vi "02 HEWH_RLTTesting_SM.vi"() -> ()   [LabVIEW 2011]
uses:
  <vilib>/Platform/fileVersionInfo.llb/FileVersionInformation.ctl
  PowerElements.ctl
  Intellifaucet/Intellfaucet Mode.ctl
  ValveBankPositions.ctl
  TestedFlowratesScenarios.ctl
  EquipReferences.ctl
  HEWH Error Enumeration.ctl
  Global HEWH.vi
panel:
  in  "Test Tank":string="101,102,103,104,105,106,107,108,109,110,111,112,113,114,115,116"
  out "Error Count":dbl
  out "result 4":bool
  out "result 3":bool
  out "result 2":bool
  out "result":bool
  out "Draws Left":i32
  out "FileNameD":path caption="FileName"
  out "FileNameC":path caption="FileName"
  out "FileNameB":path caption="FileName"
  in  "Tab Control":T1(tab)=enum."RLT Control"
  out "FileVersionInfo Out":T2
  in  "End Test":bool
  out "Finish":bool=TRUE
  out "Stop Logging":bool=TRUE
  in  "RLT Equipment":T3={"COM A"="COM3", "MW100"="MW100", "AG34970"="A-34972A", "COM B"="COM4", "COM C"="COM5", "COM D"="COM6"}
  out "Local?":bool
  out "DataQ":refnum<queue>
  in  "Flow Setting(GPM)":dbl=3.0
  in  "Temp Band":dbl=2.0
  out "Stopped Serial A":bool=TRUE
  out "Stopped Serial B":bool=TRUE
  out "Stopped Serial C":bool=TRUE
  out "Stopped Serial D":bool=TRUE
  in  "Expansion Tank?":bool=TRUE
  out "Test Started":bool=TRUE
  out "Station D Channels, Agilent":string[](array[string])
  out "Station B Channels, Agilent":string[](array[string])
  out "Station A Channels, Agilent":string[](array[string])
  out "Station C Channels, Agilent":string[](array[string])
  out "Station C Channels, MW100":string[](array[string])
  out "Station D Channels, MW100":string[](array[string])
  out "Station B Channels, MW100":string[](array[string])
  out "Station A Labels, MW100":string[](array[string])
  out "Station A Labels, Agilent":string[](array[string])
  out "Station B Labels, Agilent":string[](array[string])
  out "Station B Labels, MW100":string[](array[string])
  out "Station C Labels, Agilent":string[](array[string])
  out "Station C Labels, MW100":string[](array[string])
  out "Station D Labels, Agilent":string[](array[string])
  out "Station D Labels, MW100":string[](array[string])
  out "Station A Channels, MW100":string[](array[string])
  in  "Agilent Scan List":string="101,102,103,104,105,106,107,108,109,110,111,112,113,114,115,116"
  out "Versions":string[](array[string])
  out "Error Log":errorcluster[](array[cluster])
  in  "Gather Data Period":i32=10000
  out "Computer Name":string
  out "FileNameA":path=path "c:/data/20110112-2122_HEWH-MAN_OV.csv"
  in  "Work File Directory":path=path "c:/Work"
  out "IP Add":string
  in  "Save File Directory":path=path "c:/Data"
  in  "Divisor":i32=2000
  out "HEWH Sample Rate":i32=10
  out "T1 ComTimer":i32=1000
  in  "FlowPoll Rate":i32=10
  out "MW100 Data":dbl[](array[numeric]) format="%.4f"
  out "Agilent Output Data":dbl[](array[numeric])
  in  "MW100 Semiphore":T4=refnum
  out "Serial Data A":string[][](array[string])
  out "Serial Data B":string[][](array[string])
  out "Serial Data C":string[][](array[string])
  out "Serial Data D":string[][](array[string])
  out "A Data Array":string[][](array[string])
  out "B Data Array":string[][](array[string])
  out "C Data Array":string[][](array[string])
  out "D Data Array":string[][](array[string])
  out "# elements in queue":i32
  out "Count A":dbl
  out "Count B":dbl
  out "Count C":dbl
  out "Count D":dbl
  out "UI Update Loop":i32
  out "No Draw D":bool
  out "No Draw C":bool
  out "No Draw B":bool
  out "No Draw A":bool
  out "ComD":bool
  out "ComC":bool
  out "ComB":bool
  in  "Current Draw(D)":i32
  in  "Current Draw(C)":i32
  out "POWERC":T5
  out "POWERD":T5
  out "Alarm C":bool
  out "Alarm D":bool
  out "Alarm A":bool
  in  "Current Draw(A)":i32
  out "ComA":bool
  out "POWERA":T5
  out "POWERB":T5
  out "Alarm B":bool
  in  "Current Draw(B)":i32
  out "Drawing":bool
  in  "Start Test":bool
  in  "Num Draws (D)":i32
  in  "Num Draws (C)":i32
  in  "Num Draws (B)":i32
  out "Draw Amount (GAL)":dbl=15.0
  in  "Num Draws (A)":i32
  in  "Thermal Limit":dbl=260.0
  in  "EEV Limit":dbl=500.0
  out "Com Setting":bool=TRUE
  out "Elapsed Time":dbl format="%<%H:%M:%S>t"
  out "InitOK":bool
  out "M*(Gal)":dbl
  out "Flow":dbl=3.8899999999999997
  out "Status Message":string
  in  "Stop Test Now":bool
  out "Test States":string[](array[string])
  out "Degree Setting(F)":dbl=58.0
  out "UI":bool
  out "Tc_down":dbl
  out "Ver.":string="Development"
  in  "Pause test":bool
  out "Downspout Flow Chart":dbl(graph)=2.9
  out "Downspout Temp Chart":dbl(graph)=57.8
  out "Flow Out":dbl
  in  "K(0.2)":dbl=0.2
  out "Temp Control Sig":dbl=61.459999999999994
  out "Init Complete":bool
  out "error out":errorcluster
  # "="
  # "Gather Data Period is how often data is gathered (roughtly)\nHEWH Sample Rate is how often the serial ports are polled in GEA2.  The latest data is saved in the file.\nT1 ComTimer is the delay used through the test in the loops.\nFlow Poll Rate is how often the flow is polled (number of T1 ComTimer cycles) during Wait for Power Off."
  # "ms per cycle"
  # "HEWH RLT TEST"
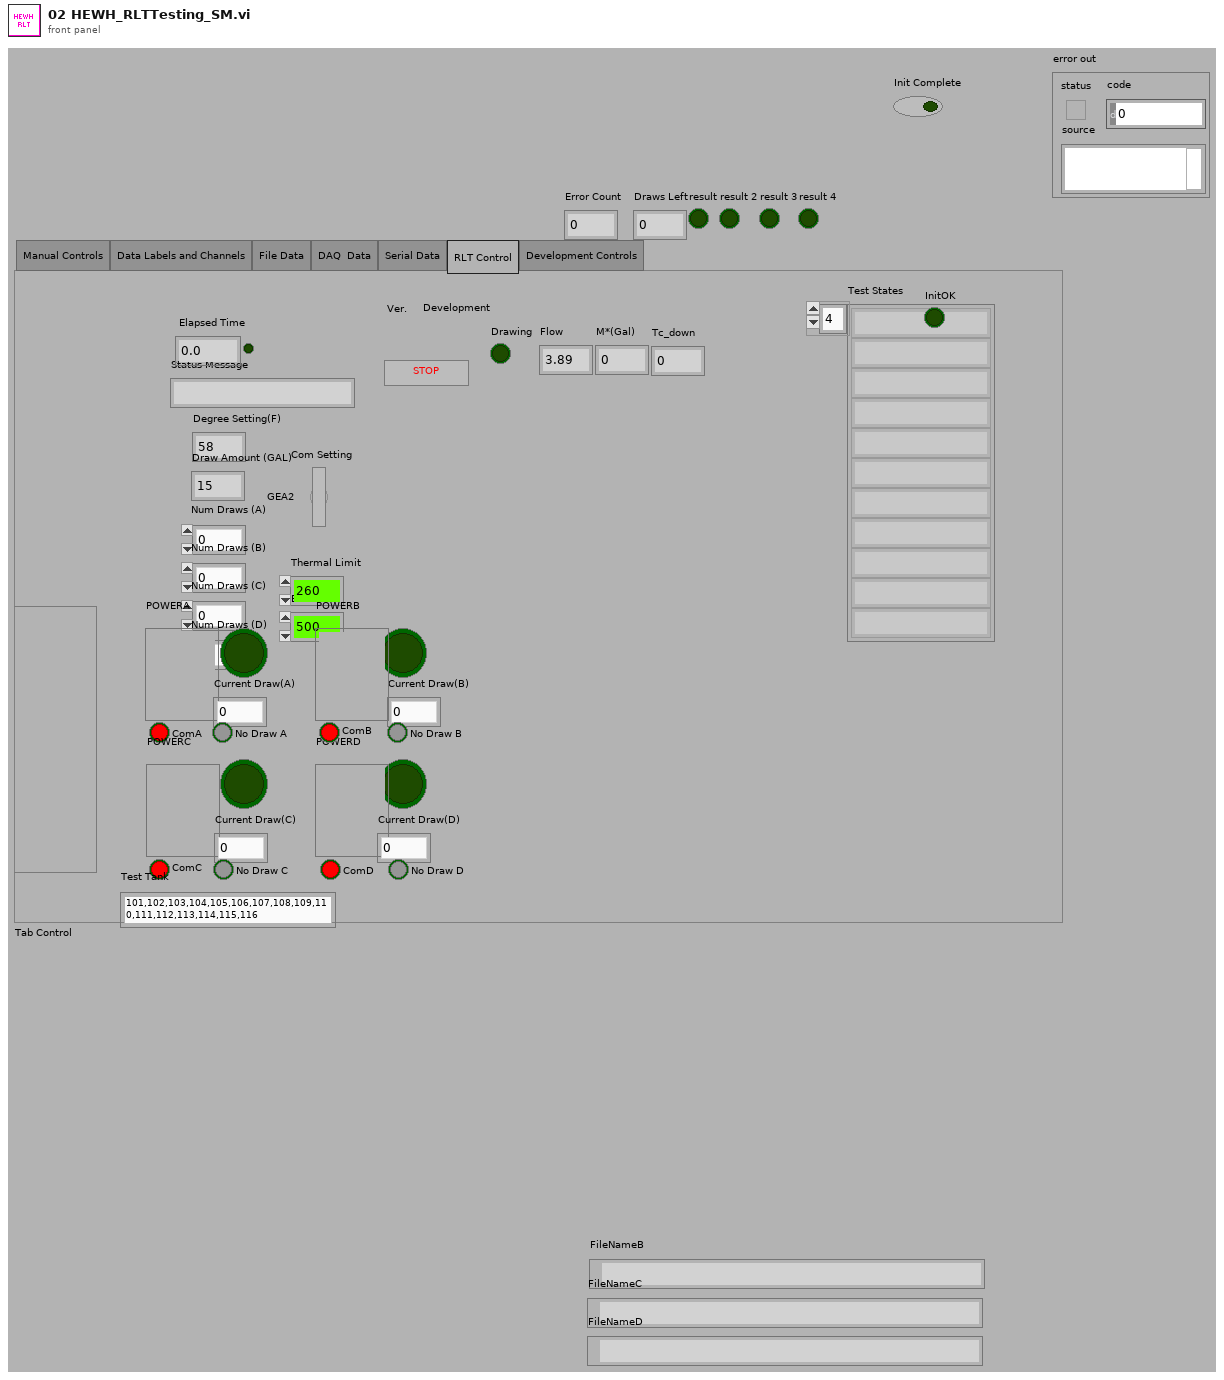
[diagram p1: front panel]
types:
  T1 = enum32{"Manual Controls", "Data Labels and Channels", "File Data", "DAQ  Data", "Serial Data", "RLT Control", "Development Controls"}
  T2 = typedef "FileVersionInformation.ctl" = cluster{"FileVersion":string, "ProductName":string, "InternalName":string, "CompanyName":string, "LegalCopyright":string, "FileDescription":string}
  T3 = cluster{"COM A":refnum<visa-resource-name>, "MW100":refnum<visa-resource-name>, "AG34970":refnum<visa-resource-name>, "COM B":refnum<visa-resource-name>, "COM C":refnum<visa-resource-name>, "COM D":refnum<visa-resource-name>}
  T4 = typedef "Semaphore RefNum" = refnum<k1>
  T5 = typedef "PowerElements.ctl" = cluster{"UE":bool, "LE":bool, "COMP":bool, "FANS":bool}
  T6 = cluster{"Degree Setting(F)":dbl, "Com Setting":bool, "EEV Limit":dbl, "Thermal Limit":dbl, "Num Draws (A)":i32, "Draw Amount (GAL)":dbl, "Num Draws (B)":i32, "Num Draws (C)":i32, "Num Draws (D)":i32}
  T7 = enum32{"invalid app kind", "Development System", "Run Time System", "Student Edition", "Embedded LabVIEW", "Evaluation", "Custom"}
  T8 = typedef "ValveBankPositions.ctl" = enum16{"Heating", "Purge", "Resting", "Draw"}
  T9 = typedef "Intellfaucet Mode.ctl" = enum16{"Adjust Temp", "Adjust Flow", "Start Flow", "Stop Flow"}
  T10 = enum32{"Invalid", "Standard", "Closed", "Hidden", "Minimized", "Maximized"}
  T11 = enum16{"Computation Start", "Computation stop", "Reset Computation", "Clear Computation"}
  T12 = typedef "TestedFlowratesScenarios.ctl" = enum16{"DRK500,Station1", "DRK375,Lab", "SRK500,Station1,5GPM FR", "DRK375,STATION3,1/2\"HOSE", "DRK500,Station1,downspout", "DRK375,Station3,thruEcocute", "DRK375,Station3,purge", "Build2,2B,Purge", "Global, Purge", "Global, Tank"}
  T13 = typedef "EquipReferences.ctl" = cluster{"COM Port":refnum<visa-resource-name>, "MW100":refnum<visa-resource-name>, "AG34970":refnum<visa-resource-name>, "Chamber":refnum<visa-resource-name>}
  T14 = typedef "HEWH Error Enumeration.ctl" = enum16{"No Error", "GEA2 Send ACK Mismatch", "GEA2 STX", "GEA2 ETX", "GEA2 CRC Mismatch", "GEA2 ReadACK", "RTD In Range Error", "Fail Mean Tank Temp", "No Flow Config Data Found", "Failed Flow During Purge", "Temp During Purge", "Confirm IF Stop Fail", "Init Draw: TC_1 Out of Range", "Flow = 0 During Draw after 20s"}
  T15 = cluster{"Core":cluster{"Current VI Reference":refnum<vi>, "Close Panel on Exit?":bool}, "RLT Equipment":cluster{"COM A":refnum<visa-resource-name>, "MW100":refnum<visa-resource-name>, "AG34970":refnum<visa-resource-name>, "COM B":refnum<visa-resource-name>, "COM C":refnum<visa-resource-name>, "COM D":refnum<visa-resource-name>}, "semaphore":T4, "Agilent Scan List":string, "Degree Setting(F)":dbl, "Flow Setting(GPM)":dbl, "Local?":bool, "Com Setting":bool, "Temp Band":dbl, "DrawsLeft":i32[], "Error Log":errorcluster[], "Test Tank":string}
  T16 = typedef "RLT Stations.ctl" = cluster{"MW100 Labels_Channels":T17[], "Agilent Labels_Channels":T17[]}
  T17 = typedef "LabelChannel.ctl" = cluster{"Label":string, "Channel":string}
  T18 = cluster{"Current VI Reference":refnum<vi>, "Close Panel on Exit?":bool}
  T19 = cluster{"MW100 Data":dbl[], "Serial Data A":string[][], "Serial Data A":string[][], "Serial Data A":string[][], "Serial Data A":string[][], "MW100 Data":dbl[]}
  T20 = cluster{"Alarm A":bool, "Current Draw(A)":i32, "ComA":bool, "POWER":T5}
  T21 = cluster{"MW100 Data":dbl[], "Serial Data A":string[][], "Serial Data B":string[][], "Serial Data C":string[][], "Serial Data D":string[][], "Agilent Output Data":dbl[]}
  T22 = cluster{"Q Element":cluster{"MW100 Data":dbl[], "Serial Data A":string[][], "Serial Data B":string[][], "Serial Data C":string[][], "Serial Data D":string[][], "Agilent Output Data":dbl[]}, "A Data Array":string[][], "B Data Array":string[][], "C Data Array":string[][], "D Data Array":string[][], "RLT Tank A":cluster{"Alarm A":bool, "Current Draw(A)":i32, "ComA":bool, "POWER":T5}, "RLT Tank B":cluster{"Alarm A":bool, "Current Draw(A)":i32, "ComA":bool, "POWER":T5}, "RLT Tank C":cluster{"Alarm A":bool, "Current Draw(A)":i32, "ComA":bool, "POWER":T5}, "RLT TankD":cluster{"Alarm A":bool, "Current Draw(A)":i32, "ComA":bool, "POWER":T5}}
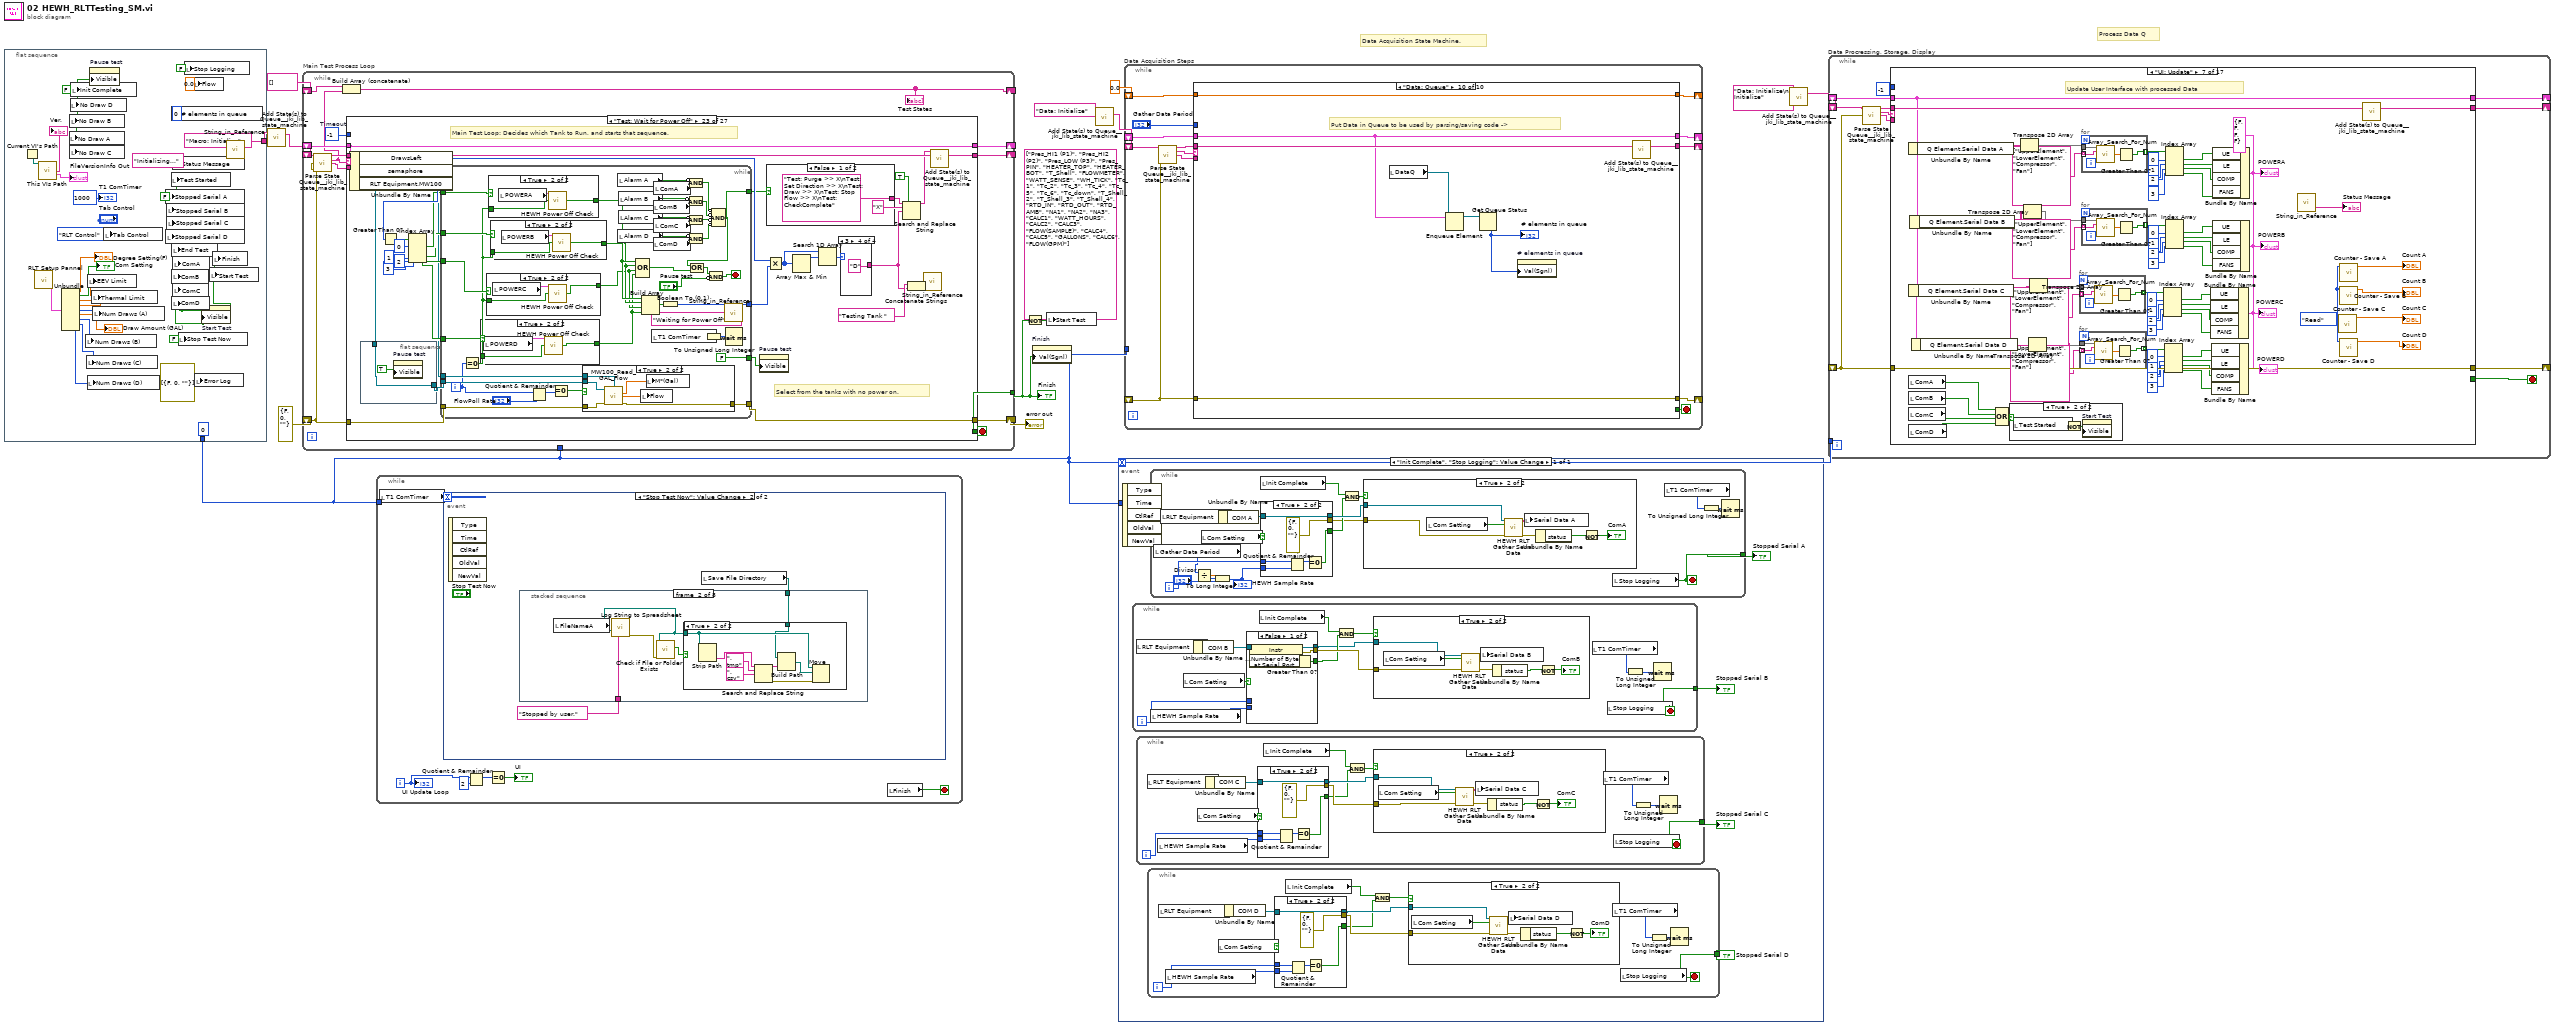
[diagram p0: block diagram]
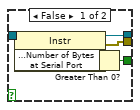
[diagram p2: hidden frame]
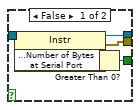
[diagram p4: hidden frame]
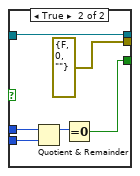
[diagram p6: hidden frame]
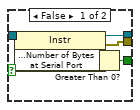
[diagram p8: hidden frame]
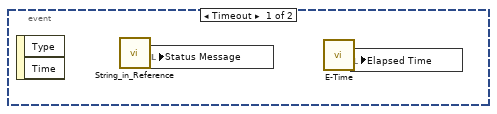
[diagram p10: hidden frame]
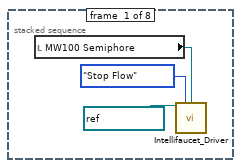
[diagram p11: hidden frame]
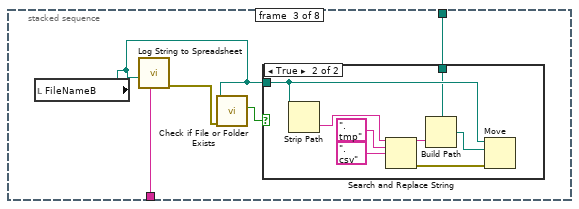
[diagram p13: hidden frame]
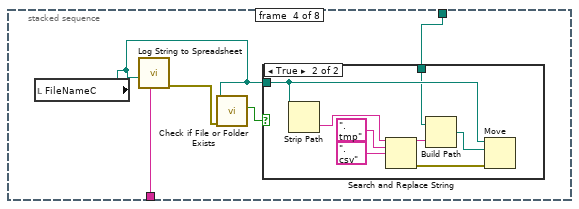
[diagram p15: hidden frame]
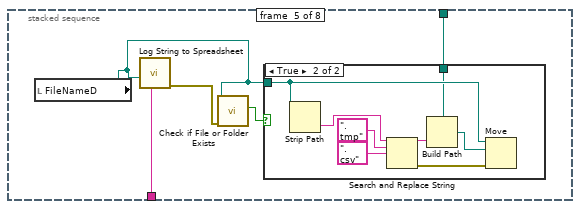
[diagram p17: hidden frame]
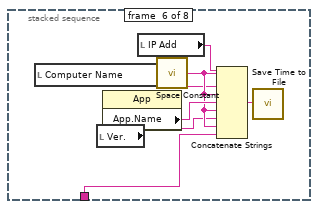
[diagram p19: hidden frame]
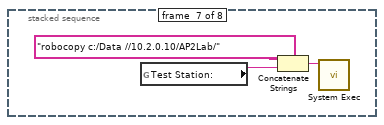
[diagram p20: hidden frame]
diagram:
  (unwired) string[] ["Pres_HI1 (P1)", "Pres_HI2 (P2)", "Pres_LOW (P3)", "Pres_PIN", "HEATER_TOP", "HEATER_BOT", "T_Shell", "FLOWMETER", "WATT_SENSE", "WH_TICK", "Tc_1", "Tc_2", "Tc_3", "Tc_4", "Tc_5", "Tc_6", "Tc_down", "T_Shell_2", "T_Shell_3", "T_Shell_4", "RTD_IN", "RTD_OUT", "RTD_AMB", "NA1", "NA2", "NA3", "CALC1", "WATT_HOURS", "CALC2", "CALC3", "FLOW(SAMPLE)", "CALC4", "CALC5", "GALLONS", "CALC6", "FLOW(GPM)"] ("output array")
  # "Process Data Q"
  # "Data Acquisition State Machine."
  n1 = flat-sequence {
    tunnel: ["Macro: Initialize"] -> w7
    tunnel: [0 ("T1 ComTimer")] -> w4
    frame #0 {
      w30 = "Initializing..." ("String")
      w14 = FALSE ("Stopped Serial A")
      w15 = FALSE ("Init Complete")
      n2 = Current VI's Path() -> (path=w18:path)
      n3 = call "RLT Setup Pannel.vi"() -> ("RLT Setup Out"=w28:T6)  [unwired: 15 in]
      n4 = call "This VIs Path.vi"("path"=w18) -> ("File Version Info"=→"Ver.":string, "FileVersionInfo Out"=→"FileVersionInfo Out":T2)  [unwired: 10 in, 3 out]
      n5 = Unbundle(w28) -> ("Degree Setting(F)"=→"Degree Setting(F)":dbl, "Com Setting"=→"Com Setting":bool, "EEV Limit"=w21:dbl, "Thermal Limit"=w20:dbl, "Num Draws (A)"=w24:i32, "Draw Amount (GAL)"=→"Draw Amount (GAL)":dbl, "Num Draws (B)"=w23:i32, "Num Draws (C)"=w22:i32, "Num Draws (D)"=w19:i32)
      n6 = local write "No Draw A"(w15) -> ()
      n7 = local write "No Draw B"(w15) -> ()
      n8 = local write "No Draw C"(w15) -> ()
      n9 = local write "No Draw D"(w15) -> ()
      n10 = local write "Init Complete"(w15) -> ()
      n11 = local write "Num Draws (B)"(w23) -> ()
      n12 = local write "Num Draws (C)"(w22) -> ()
      n13 = local write "Num Draws (D)"(w19) -> ()
      n14 = local write "EEV Limit"(w21) -> ()
      n15 = property on="Pause test" class="Bool (strict)"("Visible"=w15) -> ()  [unwired: 2 in, 2 out]
      n16 = local write "Thermal Limit"(w20) -> ()
      n17 = local write "Num Draws (A)"(w24) -> ()
      n18 = local write "Tab Control"(T1."RLT Control" ("Tab Control")) -> ()
      n19 = local write "Stopped Serial A"(w14) -> ()
      n20 = local write "Stopped Serial D"(w14) -> ()
      n21 = local write "Stopped Serial B"(w14) -> ()
      n22 = local write "Stopped Serial C"(w14) -> ()
      n23 = local write "Test Started"(w14) -> ()
      n24 = local write "# elements in queue"(0 ("# elements in queue")) -> ()
      n25 = local write "End Test"(w14) -> ()
      n26 = local write "ComB"(w14) -> ()
      n27 = local write "ComD"(w14) -> ()
      n28 = local write "Status Message"(w30) -> ()
      n29 = local write "ComA"(w14) -> ()
      n30 = local write "ComC"(w14) -> ()
      n31 = local write "Stop Test Now"(FALSE ("Stop Test Now")) -> ()
      n32 = local write "Stop Logging"(FALSE ("Stop Logging")) -> ()
      n33 = local write "Flow"(0.0 ("Flow")) -> ()
      n34 = local write "Error Log"(errorcluster[] [{"status"=FALSE, "code"=0, "source"=""}] ("Error Log")) -> ()
      n35 = property on="Start Test" class="Bool (strict)"("Visible"=w14) -> ()  [unwired: 2 in, 2 out]
      n36 = local write "Start Test"(w14) -> ()
      n37 = local write "Finish"(w14) -> ()
      n38 = call "String_in_Reference.vi"("String"=w30) -> ()  [unwired: 18 in, 1 out]
      "T1 ComTimer" <- 1000 ("T1 ComTimer")
    }
  }
  n39 = call <vilib>:"Add State(s) to Queue__jki_lib_state_machine.vi"("State(s) at Back (\"\")"=w7) -> ("States Out"=w13:string)  [unwired: 14 in]
  n40 = while "Main Test Process Loop" {
    shift-right: [w47] -> _
    shift-left: _ -> [w46]
    shift-right: [w49] -> w12
    shift-left: errorcluster {"status"=FALSE, "code"=0, "source"=""} ("Error Out") -> [w44]
    shift-right: [w48] -> _
    shift-left: w13 -> [w50]
    tunnel: [w43] -> w1
    shift-right: [w42] -> _
    shift-left: string[] [] -> [w41]
    tunnel: w4 -> [_]
    stop <- w43 stop-if-true
    w45 = -1  # Timeout
    n41 = call <vilib>:"Parse State Queue__jki_lib_state_machine.vi"("State Queue"=w50, "Error In (no error)"=w44) -> ("Remaining States"=w51:string, "Current State"=w39:string, "Arguments"=w40:string)  [unwired: 11 in]
    n42 = Build Array (concatenate)(w41, w39) -> (w42:string[])
    "Test States" <- w42
    n43 = case shown="\"Test: Wait for Power Off\"" w39 {
      selector: w39 -> [_ _ w108 _ _ _ _ _ _ _ _ _ _ _ _ _ _ _ _ _ _ w471 _ _ _ _ _]
      tunnel: w51 -> [w58 w107 w112 w130 w150 w241 w287 w306 w326 w359 w371 w390 w396 w400 w406 w412 w423 w449 w454 w465 w469 w496 w545 w634 w671 w706 w753]
      tunnel: w40 -> [_ _ _ _ _ _ _ _ _ _ _ _ _ _ _ w407 w417 _ _ _ _ _ _ w626 w666 w680 w736]
      tunnel: w46 -> [w56 w104 w110 w121 w133 w238 w275 w303 w322 w355 w368 _ w391 w397 w404 w410 w419 w446 w451 w462 w466 w489 w542 w632 w669 w704 w749]
      tunnel: [w55 w105 w114 w127 w148 w225 w267 w304 errorcluster {"status"=FALSE, "code"=0, "source"=""} ("error out") w347 w369 w380 w392 w398 w403 w408 w420 w447 w452 w463 w467 w494 w519 w618 w665 w688 w741] -> w49
      tunnel: w44 -> [w54 w105 w113 w127 w148 w239 w265 w304 w319 w356 w369 w381 w393 w398 w403 w409 w421 w447 w452 w463 w467 w494 w520 w625 w664 w691 w747]
      tunnel: [w57 w106 w111 w129 w149 w240 w286 w305 w325 w358 w370 w389 w395 w399 w405 w411 w422 w448 w453 w464 w468 w495 w544 w633 w670 w705 w752] -> w48
      tunnel: [_ _ _ _ _ _ _ _ _ TRUE _ _ _ _ _ _ _ _ _ _ _ _ _ _ _ _ _] -> w43
      tunnel: [w53 w104 w110 w128 w132 w237 w275 w303 w321 w355 w368 w388 w391 w397 w404 w410 w419 w446 w451 w462 w466 w488 w542 w632 w669 w704 w749] -> w47
      tunnel: w45 -> [w52 _ _ _ _ _ _ _ _ _ _ _ _ _ _ _ _ _ _ _ _ _ _ _ _ _ _]
      frame "", "Idle" {
        # "executes when the state queue is empty"
        n44 = event shown="[2] \"Start Test\": Value Change" {
          selector: _ -> [_ _ _ _]
          dyn-events: _ -> [_ _ _ _]
          timeout: w52 -> [_ _ _ _]
          tunnel: w58 -> [w62 w67 w86 w103]
          tunnel: [w61 w66 w85 w102] -> w57
          tunnel: w56 -> [w59 w64 w83 w100]
          tunnel: [w60 w65 w84 w101] -> w55
          tunnel: w54 -> [w60 w65 w84 w101]
          tunnel: [w59 w64 w83 w100] -> w53
          event Timeout {
            n45 = event-data() -> ()  [unwired: 1 in, 1 out]
            n46 = call <vilib>:"Add State(s) to Queue__jki_lib_state_machine.vi"("State(s) in (\"\")"=w62) -> ("States Out"=w61:string)  [unwired: 14 in]
          }
          event "End Test": Value Change {
            # "Exit Button Value Change (pressed) Event\n(this executes Macro: Exit to terminate the VI)"
            n47 = event-data() -> ()  [unwired: 1 in, 1 out]
            n48 = call <vilib>:"Add State(s) to Queue__jki_lib_state_machine.vi"("State(s) in Front (\"\")"="Macro: Exit", "State(s) in (\"\")"=w67) -> ("States Out"=w66:string)  [unwired: 13 in]
          }
          event "Start Test": Value Change {
            n49 = event-data() -> ()  [unwired: 1 in, 6 out]
            n50 = local read "Num Draws (B)"() -> (w79:i32)
            n51 = local read "Num Draws (D)"() -> (w77:i32)
            n52 = local read "Num Draws (A)"() -> (w80:i32)
            n53 = local read "Num Draws (C)"() -> (w78:i32)
            n54 = local read "FileNameD"() -> (w73:path)
            n55 = local read "FileNameC"() -> (w74:path)
            n56 = local read "FileNameA"() -> (w76:path)
            n57 = local read "FileNameB"() -> (w75:path)
            n58 = call "String_in_Reference.vi"("String"="Starting Test..." ("string")) -> ()  [unwired: 18 in, 1 out]
            n59 = Build Array(w76, w75, w74, w73) -> (w72:path[])
            n60 = Build Array(w80, w79, w78, w77) -> (w71:i32[])
            n61 = for {
              tunnel: w72 -> [w90] mode=indexing
              tunnel: w71 -> [w89] mode=indexing
              tunnel: "Start Test" -> [_]
              tunnel: [FALSE ("Visible")] -> w69
              tunnel: [TRUE] -> w68
              n62 = local read "Draw Amount (GAL)"() -> (w94:dbl)
              n63 = local read "Degree Setting(F)"() -> (w92:dbl)
              n64 = Format Into String(format string="%s %d %s %f %s %f", "Number of Draws: ", w89, " Draw Amount: ", w94, " H2O Temp In Setting: ", w92) -> (resulting string=w91:string)  [unwired: 2 in, 1 out]
              n65 = call "Log String to Spreadsheet.vi"("String"=w91, "FileName"=w90) -> ()  [unwired: 9 in, 1 out]
            }
            "Test Started" <- w68
            n66 = property on="Start Test" class="Bool (strict)"("Visible"=w69) -> ()  [unwired: 2 in, 2 out]
            n67 = call <vilib>:"Add State(s) to Queue__jki_lib_state_machine.vi"("State(s) in Front (\"\")"="Test: CheckComplete", "State(s) in (\"\")"=w86) -> ("States Out"=w85:string)  [unwired: 13 in]
          }
          event Panel Close? {
            # "Discard the event because we'll close the front panel ourselves in Macro: Exit"
            # "Close Panel button (pressed) Event\n(this executes Macro: Exit to terminate the VI)"
            n68 = event-data() -> ()  [unwired: 1 in, 1 out]
            n69 = call <vilib>:"Add State(s) to Queue__jki_lib_state_machine.vi"("State(s) in Front (\"\")"="Macro: Exit", "State(s) in (\"\")"=w103) -> ("States Out"=w102:string)  [unwired: 13 in]
            n70 = event-data("Discard?"=TRUE) -> ()  [unwired: 1 in, 1 out]
          }
        }
      }
      frame "---------- Core ----------" {
        # "Do not put any code in this frame.\n(it is a separator no-op)"
        n71 = call <vilib>:"Add State(s) to Queue__jki_lib_state_machine.vi"("State(s) in (\"\")"=w107) -> ("States Out"=w106:string)  [unwired: 14 in]
      }
      frame Default {
        w117 = 42 items=["No error", "Argument error", "Memory is full", "Out of zone", "End of file", "File already open", "Generic file I/O error", "File not found", "File permission error", "Disk is full", "Duplicate path", "Too many files open", "System feature not enabled", "Resource file not found", "Cannot add resource", "Resource not found", "Image not found", "Image memory error", "Pen does not exist", "Config type invalid", "Config token not found", "Config parse error", "Config memory error", "Bad external code format", "Bad external code offset", "External code not present", "Null window", "Destroy window error", "Null menu", "Print aborted", "Bad print record", "Print driver error", "Windows error during printing", "Memory error during printing", "Print dialog error", "Generic print error", "Invalid device refnum", "Device not found", "Device parameter error", "Device unit error", "Cannot open device", "Device call aborted", "Generic error", "Cancelled by user", "Object ID too low", "Object ID too high", "Object not in heap", "Unknown heap", "Unknown object (invalid DefProc)", "Unknown object (DefProc not in table)", "Message out of range", "Invalid (null) method", "Unknown message", "Manager call not supported", "Bad address", "Network operation in progress", "Network operation timed out", "Connection is busy", "Network attribute not supported", "Network error", "Address in use", "System out of memory", "Connection aborted", "Connection refused", "Not connected", "Already connected", "Connection closed", "Initialization error (interapplication manager)", "Bad occurrence", "Wait on unbound occurrence handler", "Occurrence queue overflow", "Datalog type conflict", "Unused", "Unrecognized type (interapplication manager)", "Memory corrupt", "Failed to make temporary DLL", "Old CIN version", "Drag socket not found", "Failed to load drop-object", "Failed to register OLE object", "Failed to release OLE object", "Format specifier type mismatch", "Unknown format specifier", "Too few format specifiers", "Too many format specifiers", "Scan failed", "Newer CIN version", "Error converting to variant", "Runtime menu error", "Password tampered", "Variant attribute not found", "Incompatible variant data type", "Event data is not available", "Event Store is not present", "Occurrence is not found", "Event Queue is not created", "Event info is not available", "Refnum passed is NULL", "Error retrieving Class GUID", "Error retrieving CoClass GUID", "Error retrieving TypeLib GUID.", "Bad built application magic bytes.", "Specific driver is different from the specific driver associated with the Logical Name.", "There is no session opened to the class driver.", "Max Error", "MAX - Error with config objects", "MAX - Error loading configuration", "MAX - Group not supported"]
        # "Current State"
        # "Do not delete, rename, or modify this frame.\n(this is used to capture unhandled states and typos)"
        # "Handle mistyped state name (developer tool)"
        n72 = Format Into String(format string="Software Exception: Unhandled State \"%s\"." ("message"), error in=w113, w108) -> (resulting string=w116:string, error out=w115:errorcluster)  [unwired: 1 in]
        n73 = call <vilib>:"Error Cluster From Error Code.vi"("show call chain? (False)"=TRUE, "error in (no error)"=w115, "error message (\"\")"=w116, "error code (0)"=w117) -> ("error out"=w114:errorcluster)  [unwired: 5 in]
        n74 = call <vilib>:"Add State(s) to Queue__jki_lib_state_machine.vi"("State(s) in (\"\")"=w112) -> ("States Out"=w111:string)  [unwired: 14 in]
      }
      frame "Initialize Core Data" {
        # "Do not delete, rename, or modify this frame.\n(this is used to determine panel behavior on exit)"
        # "originally closed?"
        # "exe?"
        # "If panel starts closed or is an EXE, then close it when we exit"
        n75 = property class="VI"() -> ("Front Panel.Open"=w126:bool)  [unwired: 2 in, 2 out]
        n76 = property class="App"() -> ("App.Kind"=w125:T7)  [unwired: 2 in, 2 out]
        n77 = control-ref of="Current VI Reference"() -> (w119:refnum<vi>)
        n78 = Not(x=w126) -> (.not. x?=w123:bool)
        n79 = Equal?(x=w125, y=T7."Run Time System" ("Application:Kind")) -> (x = y?=w122:bool)
        n80 = Or(x=w123, y=w122) -> (x .or. y?=w120:bool)
        n81 = Bundle By Name(cluster=w121, "Core.Current VI Reference"=w119, "Core.Close Panel on Exit?"=w120) -> (w128:T15)
        n82 = call <vilib>:"Add State(s) to Queue__jki_lib_state_machine.vi"("State(s) in (\"\")"=w130) -> ("States Out"=w129:string)  [unwired: 14 in]
      }
      frame "Initialize Channels" {
        (unwired) string[][] [["Pres_HI1 (P1)", "Pres_HI2 (P2)", "Pres_LOW (P3)", "HEATER_TOP", "HEATER_BOT", "T_Shell", "Tc_1", "Tc_2", "Tc_3", "Tc_4", "Tc_5", "Tc_6", "Tc_down", "T_Shell_2", "T_Shell_3", "T_Shell_4", "RTD_IN", "RTD_OUT", "RTD_AMB", "WATT_HOURS", "GALLONS", "FLOW(GPM)"], ["011", "012", "013", "015", "016", "017", "021", "022", "023", "024", "025", "026", "027", "028", "029", "030", "031", "032", "033", "A002", "A008", "A010"]] ("MW100 Labels and Chanels")
        # "Gallons must be first, all others are checked using thermal limit."
        n83 = call "HEWH Channel Test Labels for RLT.vi"() -> ("Station A"=w147:T16, "Station B"=w146:T16, "Station C"=w145:T16, "Station D"=w144:T16)  [unwired: 12 in]
        n84 = Unbundle By Name(w147) -> ("MW100 Labels_Channels"=w143:T17[], "Agilent Labels_Channels"=w142:T17[])
        n85 = Unbundle By Name(w146) -> ("MW100 Labels_Channels"=w141:T17[], "Agilent Labels_Channels"=w140:T17[])
        n86 = Unbundle By Name(w144) -> ("MW100 Labels_Channels"=w136:T17[], "Agilent Labels_Channels"=w137:T17[])
        n87 = Unbundle By Name(w145) -> ("MW100 Labels_Channels"=w139:T17[], "Agilent Labels_Channels"=w138:T17[])
        n88 = stacked-sequence {
          tunnel: w143 -> [w160 _ _ _ _]
          tunnel: w142 -> [w158 _ _ _ _]
          tunnel: w141 -> [_ w174 _ _ _]
          tunnel: w140 -> [_ w173 _ _ _]
          tunnel: w139 -> [_ _ w190 _ _]
          tunnel: w138 -> [_ _ w189 _ _]
          tunnel: w137 -> [_ _ _ w206 _]
          tunnel: w136 -> [_ _ _ w205 _]
          tunnel: string[] ["A008", "A010", "033", "027"] -> [w151 w167 w183 w200 _]
          tunnel: string[] ["GALLONS", "FLOW(GPM)", "RTD_AMB", "Tc_down"] -> [w152 w168 w184 w199 _]
          tunnel: [_ _ _ _ w215] -> w131
          frame #0 {
            n89 = for {
              tunnel: w160 -> [w166] mode=indexing
              tunnel: [w165] -> w159 mode=indexing
              tunnel: [w164] -> w156 mode=indexing
              n90 = Unbundle By Name(w166) -> ("Label"=w165:string, "Channel"=w164:string)
            }
            n91 = for {
              tunnel: w158 -> [w163] mode=indexing
              tunnel: [w162] -> w157 mode=indexing
              tunnel: [w161] -> w155 mode=indexing
              n92 = Unbundle By Name(w163) -> ("Label"=w162:string, "Channel"=w161:string)
            }
            "Station A Labels, Agilent" <- w157
            "Station A Channels, Agilent" <- w155
            n93 = Build Array (concatenate)(w151, w156) -> (→"Station A Channels, MW100":string[])
            n94 = Build Array (concatenate)(w152, w159) -> (→"Station A Labels, MW100":string[])
          }
          frame #1 {
            n95 = for {
              tunnel: [w182] -> w176 mode=indexing
              tunnel: w174 -> [w181] mode=indexing
              tunnel: [w180] -> w172 mode=indexing
              n96 = Unbundle By Name(w181) -> ("Label"=w182:string, "Channel"=w180:string)
            }
            n97 = for {
              tunnel: [w179] -> w175 mode=indexing
              tunnel: w173 -> [w178] mode=indexing
              tunnel: [w177] -> w171 mode=indexing
              n98 = Unbundle By Name(w178) -> ("Label"=w179:string, "Channel"=w177:string)
            }
            "Station B Labels, Agilent" <- w175
            "Station B Channels, Agilent" <- w171
            n99 = Build Array (concatenate)(w168, w176) -> (→"Station B Labels, MW100":string[])
            n100 = Build Array (concatenate)(w167, w172) -> (→"Station B Channels, MW100":string[])
          }
          frame #2 {
            n101 = for {
              tunnel: [w198] -> w192 mode=indexing
              tunnel: w190 -> [w197] mode=indexing
              tunnel: [w196] -> w188 mode=indexing
              n102 = Unbundle By Name(w197) -> ("Label"=w198:string, "Channel"=w196:string)
            }
            n103 = for {
              tunnel: [w195] -> w191 mode=indexing
              tunnel: w189 -> [w194] mode=indexing
              tunnel: [w193] -> w187 mode=indexing
              n104 = Unbundle By Name(w194) -> ("Label"=w195:string, "Channel"=w193:string)
            }
            "Station C Labels, Agilent" <- w191
            "Station C Channels, Agilent" <- w187
            n105 = Build Array (concatenate)(w184, w192) -> (→"Station C Labels, MW100":string[])
            n106 = Build Array (concatenate)(w183, w188) -> (→"Station C Channels, MW100":string[])
          }
          frame #3 {
            n107 = for {
              tunnel: [w211] -> w207 mode=indexing
              tunnel: w206 -> [w210] mode=indexing
              tunnel: [w209] -> w203 mode=indexing
              n108 = Unbundle By Name(w210) -> ("Label"=w211:string, "Channel"=w209:string)
            }
            "Station D Labels, Agilent" <- w207
            "Station D Channels, Agilent" <- w203
            n109 = for {
              tunnel: [w214] -> w208 mode=indexing
              tunnel: w205 -> [w213] mode=indexing
              tunnel: [w212] -> w204 mode=indexing
              n110 = Unbundle By Name(w213) -> ("Label"=w214:string, "Channel"=w212:string)
            }
            n111 = Build Array (concatenate)(w199, w208) -> (→"Station D Labels, MW100":string[])
            n112 = Build Array (concatenate)(w200, w204) -> (→"Station D Channels, MW100":string[])
          }
          frame #4 {
            n113 = local read "Station A Channels, Agilent"() -> (w223:string[])
            n114 = local read "Station B Channels, Agilent"() -> (w220:string[])
            n115 = local read "Station C Channels, Agilent"() -> (w221:string[])
            n116 = local read "Station D Channels, Agilent"() -> (w222:string[])
            n117 = Build Array (concatenate)(w223, w220, w221, w222) -> (w219:string[])
            n118 = Array To Spreadsheet String(delimiter (Tab)="," ("format string"), array=w219, 3:"%s" ("format string")) -> (spreadsheet string=w216:string)
            n119 = call <vilib>:"Trim Whitespace.vi"("string"=w216) -> ("trimmed string"=w215:string)  [unwired: 1 in]
          }
        }
        n120 = call <vilib>:"Add State(s) to Queue__jki_lib_state_machine.vi"("State(s) in (\"\")"=w150) -> ("States Out"=w149:string)  [unwired: 14 in]
        n121 = Bundle By Name(cluster=w133, "Agilent Scan List"=w131) -> (w132:T15)
        n122 = local write "Agilent Scan List"(w131) -> ()
      }
      frame "Initialize Equipment" {
        w231 = u16[] [0, 1, 2, 3] items=["A", "B", "C", "D"]
        n123 = Unbundle By Name(w238) -> ("RLT Equipment"=w236:T3, "semaphore"=w230:T4, "Local?"=w235:bool, "Com Setting"=w234:bool, "Agilent Scan List"=w233:string)
        n124 = local write "Agilent Scan List"(w233) -> ()
        n125 = case shown="True" w235 {
          tunnel: w239 -> [w252 w262]
          tunnel: [w252 w261] -> w232
          tunnel: w236 -> [w251 w255]
          tunnel: [w251 w259] -> w229
          tunnel: w230 -> [_ w260]
          tunnel: w233 -> [_ w256]
          tunnel: w234 -> [_ w253]
          frame False {
          }
          frame True {
            n126 = call "HEWH Init_RLT_Equip.vi"("Semiphore"=w260, "Error In"=w262, "GEA?"=w253, "Agilent Channel Input"=w256, "RLT Equipment"=w255) -> ("Error Out"=w261:errorcluster, "Computer Name"=→"Computer Name":string, "LAN IP Address"=→"IP Add":string, "RLT Equipment Out"=w259:T3, "InitOK"=→"InitOK":bool)  [unwired: 2 in]
          }
        }
        n127 = local write "MW100 Semiphore"(w230) -> ()
        n128 = Unbundle By Name(w229) -> ("MW100"=w228:refnum<visa-resource-name>)
        n129 = local write "RLT Equipment"(w229) -> ()
        n130 = Bundle By Name(cluster=w238, "RLT Equipment"=w229, "semaphore"=w230) -> (w237:T15)
        n131 = for {
          tunnel: [w250] -> w225
          tunnel: w232 -> [w249]
          tunnel: w231 -> [w248] mode=indexing
          tunnel: w230 -> [w247]
          tunnel: w228 -> [w246]
          tunnel: "Expansion Tank?" -> [w245]
          tunnel: ValveBankPositions."Heating" ("Valve Bank Setting") -> [w244]
          n132 = call "HEWH Set Valves.vi"("VISA session"=w246, "Valve Bank"=w248, "Semiphore"=w247, "Expansion Tank?"=w245, "Valve Bank Setting"=w244, "Error In"=w249) -> ("Error Out"=w250:errorcluster)  [unwired: 8 in, 1 out]
        }
        n133 = case shown="Error" w225 {
          tunnel: ["" ("State(s) in Front (\"\")") "Exit" ("State(s) in Front (\"\")")] -> w224
          frame No Error {
          }
          frame Error {
          }
        }
        n134 = call <vilib>:"Add State(s) to Queue__jki_lib_state_machine.vi"("State(s) in Front (\"\")"=w224, "State(s) in (\"\")"=w241) -> ("States Out"=w240:string)  [unwired: 13 in]
      }
      frame "Initialize Files" {
        # "Do not put any code in this frame.\n(it is a separator no-op)"
        n135 = Unbundle By Name(w275) -> ("RLT Equipment.COM A"=w274:refnum<visa-resource-name>, "RLT Equipment.COM B"=w273:refnum<visa-resource-name>, "RLT Equipment.COM C"=w272:refnum<visa-resource-name>, "RLT Equipment.COM D"=w271:refnum<visa-resource-name>)
        n136 = local read "FileVersionInfo Out"() -> (w264:T2)
        n137 = call "HEWH Config Read.vi"("error in (no error)"=w265) -> ("error out"=w268:errorcluster)  [unwired: 13 in, 1 out]
        n138 = Build Array(w274, w273, w272, w271) -> (w270:refnum<visa-resource-name>[])
        n139 = local read "Computer Name"() -> (w281:string)
        n140 = Unbundle By Name(w264) -> ("ProductName"=w283:string, "FileVersion"=w282:string)
        n141 = call "Data_File_Init RLT.vi"("Data Directory In:"="Work File Directory", "Ambient Temp,RH:"=w283, "Version In:"=w282, "Computer Name In:"=w281, "error in (no error)"=w268, "File Extension:"="tmp") -> ("FileNameA"=w280:path, "FileNameB"=w279:path, "FileNameC"=w278:path, "FileNameD"=w277:path, "error out"=w266:errorcluster)  [unwired: 5 in]
        "FileNameA" <- w280
        "FileNameB" <- w279
        "FileNameC" <- w278
        "FileNameD" <- w277
        n142 = local read "Com Setting"() -> (w263:bool)
        n143 = Build Array(w280, w279, w278, w277) -> (w276:path[])
        n144 = case shown="False" w263 {
          tunnel: w276 -> [_ w293]
          tunnel: w270 -> [_ w292]
          tunnel: [w288 w290] -> w267
          tunnel: w266 -> [w288 w289]
          frame False {
          }
          frame True {
            n145 = for {
              tunnel: w293 -> [w298] mode=indexing
              shift-right: [w294] -> w290
              shift-left: w289 -> [w294]
              tunnel: w292 -> [w296] mode=indexing
              tunnel: [w295] -> w291 mode=indexing
              n146 = call "GEA2_RQST_SOFTWARE_VER.vi"("ComPort"=w296) -> ("Software Version"=w295:string, "Error Out"=w297:errorcluster)  [unwired: 11 in, 2 out]
              n147 = call "Log String to Spreadsheet.vi"("String"=w295, "error in (no error)"=w297, "FileName"=w298) -> ()  [unwired: 8 in, 1 out]
            }
            "Versions" <- w291
          }
        }
        n148 = case shown="Error" w267 {
          tunnel: ["" ("State(s) in Front (\"\")") "Exit" ("State(s) in Front (\"\")")] -> w269
          frame No Error {
          }
          frame Error {
          }
        }
        n149 = call <vilib>:"Add State(s) to Queue__jki_lib_state_machine.vi"("State(s) in Front (\"\")"=w269, "State(s) in (\"\")"=w287) -> ("States Out"=w286:string)  [unwired: 13 in]
      }
      frame "Init Complete" {
        w302 = TRUE ("Init Complete")
        n150 = flat-sequence {
          frame #0 {
            n151 = local read "Computer Name"() -> (w307:string)
            n152 = local read "Ver."() -> (w308:string)
            n153 = property class="App"() -> ("App.Name"=w311:string)  [unwired: 2 in, 2 out]
            n154 = local read "IP Add"() -> (w312:string)
            n155 = call <vilib>:"Space Constant.vi"() -> ("String"=w310:string)
            n156 = Concatenate Strings(w312, w310, w307, w310, w311, w310, w308, w310, "Started." ("string")) -> (w313:string)
            n157 = call "Save Time to File.vi"("String"=w313) -> ()  [unwired: 13 in, 2 out]
          }
          frame #1 {
            n158 = disable-structure shown="Enabled" {
              frame Disabled {
                n159 = global read "Global HEWH.vi" "Test Station:"() -> (w315:string)
                n160 = Concatenate Strings("robocopy c:/Data //10.2.0.10/AP2Lab/" ("command line"), w315) -> (w314:string)
                n161 = call <vilib>:"System Exec.vi"("command line"=w314) -> ()  [unwired: 7 in, 4 out]
              }
              frame Enabled {
              }
            }
          }
        }
        n162 = property on="Init Complete" class="Bool (strict)"("Val(Sgnl)"=w302) -> ()  [unwired: 2 in, 2 out]
        n163 = call "String_in_Reference.vi"("String"="Init Complete") -> ()  [unwired: 18 in, 1 out]
        n164 = call <vilib>:"Add State(s) to Queue__jki_lib_state_machine.vi"("State(s) in (\"\")"=w306) -> ("States Out"=w305:string)  [unwired: 14 in]
        "Init Complete" <- w302
      }
      frame "Error Handler" {
        # "Unhandled Error -- Display it"
        # "Handle any errors here.\nYou can also output any states to clean-up after errors occur"
        # "Clear error"
        n165 = Unbundle By Name(w322) -> ("Error Log"=w323:errorcluster[])
        n166 = local read "Init Complete"() -> (w318:bool)
        n167 = Build Array (concatenate)(w323, w319) -> (w320:errorcluster[])
        n168 = case shown="True" w318 {
          tunnel: w320 -> [_ w344]
          tunnel: w319 -> [w328 w343]
          tunnel: ["Exit" ""] -> w317
          frame False {
            n169 = call <vilib>:"Simple Error Handler.vi"("error in (no error)"=w328) -> ()  [unwired: 4 in, 5 out]
          }
          frame True {
            n170 = call "Counter.vi"() -> ("Count"=w341:dbl)  [unwired: 11 in]
            "Error Count" <- w341
            n171 = Unbundle By Name(w343) -> ("code"=w336:i32, "source"=w337:string)  [unwired: 1 out]
            n172 = local read "FileNameC"() -> (w333:path)
            n173 = local read "FileNameC"() -> (w332:path)
            n174 = local read "FileNameA"() -> (w335:path)
            n175 = local read "FileNameB"() -> (w334:path)
            n176 = Format Into String(format string="%s %d %s %d %s %s", "Error Count: " ("input 1"), w341, " Code: " ("input 1"), w336, " Source: " ("input 1"), w337) -> (resulting string=w330:string)  [unwired: 2 in, 1 out]
            n177 = Build Array(w335, w334, w333, w332) -> (w331:path[])
            n178 = for {
              tunnel: w331 -> [w346] mode=indexing
              tunnel: w330 -> [w345]
              n179 = call "Log String to Spreadsheet.vi"("String"=w345, "FileName"=w346) -> ()  [unwired: 9 in, 1 out]
            }
            "Error Log" <- w344
          }
        }
        n180 = Bundle By Name(cluster=w322, "Error Log"=w320) -> (w321:T15)
        n181 = call <vilib>:"Add State(s) to Queue__jki_lib_state_machine.vi"("State(s) in Front (\"\")"=w317, "State(s) in (\"\")"=w326) -> ("States Out"=w325:string)  [unwired: 13 in]
      }
      frame "Exit" {
        w349 = u16[] [0, 1, 2, 3] items=["A", "B", "C", "D"]
        # "Do not put any code in this frame.\n(No errors that occur here will be handled.)"
        n182 = Unbundle By Name(w355) -> ("semaphore"=w350:T4, "RLT Equipment.MW100"=w354:refnum<visa-resource-name>)
        n183 = call "Intellifaucet_Driver.vi"("VISA session"=w354, "Mode"=Intellfaucet_Mode."Stop Flow", "Semiphore"=w350, "Error In"=w356) -> ("VISA session out"=w351:refnum<visa-resource-name>, "Error Out"=w352:errorcluster)  [unwired: 10 in]
        n184 = for {
          tunnel: w351 -> [w366]
          tunnel: w350 -> [w365]
          tunnel: w349 -> [w361] mode=indexing
          shift-right: [w360] -> w347
          shift-left: w352 -> [w367]
          n185 = call "Solenoid Bank.vi"("VISA session"=w366, "Semiphore"=w365, "Valve Bank"=w361, "Drain Valve"=enum8{"OPEN", "CLOSE"}."CLOSE", "Output Valve"=enum8{"CLOSE", "OPEN"}."OPEN", "Input Valve"=enum8{"OPEN", "CLOSE"}."CLOSE", "Error In"=w367) -> ("Error Out"=w360:errorcluster)  [unwired: 7 in, 1 out]
        }
        n186 = call "String_in_Reference.vi"("String"="Stopping Test..." ("string")) -> ()  [unwired: 18 in, 1 out]
        n187 = call <vilib>:"Add State(s) to Queue__jki_lib_state_machine.vi"("State(s) in (\"\")"=w359) -> ("States Out"=w358:string)  [unwired: 14 in]
      }
      frame "---------- Data ----------" {
        # "Do not put any code in this frame.\n(It is a separator no-op. You can make a copy of this frame to create a new Data frame)"
        n188 = call <vilib>:"Add State(s) to Queue__jki_lib_state_machine.vi"("State(s) in (\"\")"=w371) -> ("States Out"=w370:string)  [unwired: 14 in]
      }
      frame "Data: Initialize" {
        w375 = errorcluster[] []  # Error Log
        w377 = i32[] []  # DrawsLeft
        w378 = 0 ("Current Draw(D)")
        w387 = T18 {"Current VI Reference"=refnum, "Close Panel on Exit?"=FALSE}  # Core
        # "Initialize the shift-register data, here.\n(data names are defined by what you wire into the bundle function)"
        n189 = local read "Degree Setting(F)"() -> (w373:dbl)
        n190 = local read "Com Setting"() -> (w374:bool)
        n191 = call "Semiphore-Create-Local.vi"("Semiphore"="MW100 Semiphore", "error in (no error)"=w381) -> ("semaphore"=w376:T4, "Local?"=w383:bool, "error out"=w380:errorcluster)  [unwired: 15 in]
        "Local?" <- w383
        n192 = local write "MW100 Semiphore"(w376) -> ()
        n193 = Bundle("Core"=w387, "RLT Equipment"="RLT Equipment", "semaphore"=w376, "Agilent Scan List"="Agilent Scan List", "Degree Setting(F)"=w373, "Flow Setting(GPM)"="Flow Setting(GPM)", "Local?"=w383, "Com Setting"=w374, "Temp Band"="Temp Band", "DrawsLeft"=w377, "Error Log"=w375, "Test Tank"="Test Tank") -> (w388:T15)  [unwired: 1 in]
        n194 = call <vilib>:"Add State(s) to Queue__jki_lib_state_machine.vi"("State(s) in (\"\")"=w390) -> ("States Out"=w389:string)  [unwired: 14 in]
        n195 = local write "Current Draw(D)"(w378) -> ()
        n196 = local write "Current Draw(C)"(w378) -> ()
        n197 = local write "Current Draw(A)"(w378) -> ()
        n198 = local write "Current Draw(B)"(w378) -> ()
      }
      frame "Data: Cleanup" {
        # "Cleanup any data and references, here.\n(this is called automatically, by the Macro: Exit)"
        n199 = Unbundle By Name(w391) -> ("Core.Current VI Reference"=w394:refnum<vi>)
        n200 = Close Reference(reference=w394, error in (no error)=w393) -> (error out=w392:errorcluster)
        n201 = call <vilib>:"Add State(s) to Queue__jki_lib_state_machine.vi"("State(s) in (\"\")"=w396) -> ("States Out"=w395:string)  [unwired: 14 in]
      }
      frame "---------- UI ----------" {
        # "Do not put any code in this frame.\n(It is a separator no-op. You can make a copy of this frame to create a new UI frame)"
        n202 = call <vilib>:"Add State(s) to Queue__jki_lib_state_machine.vi"("State(s) in (\"\")"=w400) -> ("States Out"=w399:string)  [unwired: 14 in]
      }
      frame "UI: Initialize" {
        w401 = FALSE ("Blinking")
        w402 = FALSE ("Recording Data")
        # "Initialize the User Interface, here.\n(this is called automatically, by the Macro: Init)"
        n203 = property on="Current Draw(A)" class="DigNum (strict)"("Blinking"=w401) -> ()  [unwired: 2 in, 2 out]
        n204 = property on="Current Draw(B)" class="DigNum (strict)"("Blinking"=w401) -> ()  [unwired: 2 in, 2 out]
        n205 = property on="Current Draw(D)" class="DigNum (strict)"("Blinking"=w401) -> ()  [unwired: 2 in, 2 out]
        n206 = property on="Current Draw(C)" class="DigNum (strict)"("Blinking"=w401) -> ()  [unwired: 2 in, 2 out]
        n207 = local write "Init Complete"(w402) -> ()
        n208 = local write "Alarm A"(w402) -> ()
        n209 = local write "Alarm D"(w402) -> ()
        n210 = local write "Alarm B"(w402) -> ()
        n211 = local write "Alarm C"(w402) -> ()
        n212 = local write "Finish"(w402) -> ()
        n213 = call <vilib>:"Add State(s) to Queue__jki_lib_state_machine.vi"("State(s) in (\"\")"=w406) -> ("States Out"=w405:string)  [unwired: 14 in]
      }
      frame "UI: Cursor Set" {
        # "Argument"
        # "Set and Unset Cursor Busy.\n(Usage: \"UI: Cursor Set >> Busy|Idle\")"
        n214 = case shown="\"Busy\"" w407 {
          tunnel: w409 -> [w414 w416]
          tunnel: [w413 w415] -> w408
          frame "Idle", Default {
            n215 = call <vilib>:"Unset Busy.vi"("error in (no error)"=w414) -> ("error out"=w413:errorcluster)  [unwired: 10 in]
          }
          frame "Busy" {
            n216 = call <vilib>:"Set Busy.vi"("error in (no error)"=w416) -> ("error out"=w415:errorcluster)  [unwired: 9 in, 1 out]
          }
        }
        n217 = call <vilib>:"Add State(s) to Queue__jki_lib_state_machine.vi"("State(s) in (\"\")"=w412) -> ("States Out"=w411:string)  [unwired: 14 in]
      }
      frame "UI: Front Panel State" {
        # "Argument"
        # "Set Front Panel Open or Closed\n(Usage: \"UI: Front Panel State >> Open|Close\")"
        n218 = Unbundle By Name(w419) -> ("Core.Current VI Reference"=w418:refnum<vi>)
        n219 = case shown="\"Open\", Default" w417 {
          tunnel: w421 -> [w427 w440]
          tunnel: [w429 w441] -> w420
          tunnel: w418 -> [w428 w438]
          frame "Open", Default {
            n220 = property class="VI"(reference=w428, error in=w427) -> (reference out=w425:refnum<vi>, error out=w426:errorcluster, "Front Panel.Open"=w424:bool)
            n221 = case shown="False" w424 {
              tunnel: [w432 w435] -> w429
              tunnel: w426 -> [w431 w435]
              tunnel: w425 -> [w430 _]
              frame False {
                n222 = invoke class="VI" method="FP.Open"(reference=w430, error in=w431, "Activate"=TRUE, "State"=T10."Standard") -> (error out=w432:errorcluster)  [unwired: 1 in, 4 out]
              }
              frame True {
              }
            }
          }
          frame "Close" {
            n223 = property class="VI"(reference=w438, error in=w440) -> (reference out=w437:refnum<vi>, error out=w439:errorcluster, "Front Panel.Open"=w436:bool)
            n224 = case shown="True" w436 {
              tunnel: [w442 w445] -> w441
              tunnel: w439 -> [w442 w444]
              tunnel: w437 -> [_ w443]
              frame False {
              }
              frame True {
                n225 = invoke class="VI" method="FP.Close"(reference=w443, error in=w444) -> (error out=w445:errorcluster)  [unwired: 1 in, 2 out]
              }
            }
          }
        }
        n226 = call <vilib>:"Add State(s) to Queue__jki_lib_state_machine.vi"("State(s) in (\"\")"=w423) -> ("States Out"=w422:string)  [unwired: 14 in]
      }
      frame "---------- Macro ----------" {
        # "Do not put any code in this frame.\n(It is a separator no-op. You can make a copy of this frame to create a new Macro frame)"
        n227 = call <vilib>:"Add State(s) to Queue__jki_lib_state_machine.vi"("State(s) in (\"\")"=w449) -> ("States Out"=w448:string)  [unwired: 14 in]
      }
      frame "Macro: Initialize" {
        w450 = "Data: Initialize\nInitialize Core Data\nUI: Initialize\nUI: Front Panel State >> Open\nInitialize Channels\nInitialize Equipment\nInitialize Files\nInit Complete"  # Data: Initialize Initialize Core Data UI: Initialize UI: Front Panel State >> Open Initialize Channels Initialize Equipment Initialize Files Init Complete
        # "Initialization Macro\n(This is called once, when the VI starts)"
        n228 = call <vilib>:"Add State(s) to Queue__jki_lib_state_machine.vi"("State(s) in Front (\"\")"=w450, "State(s) in (\"\")"=w454) -> ("States Out"=w453:string)  [unwired: 13 in]
      }
      frame "Macro: Exit" {
        # "Exit Macro\n(This is called once, when the VI exits)"
        n229 = Unbundle By Name(w462) -> ("Core.Close Panel on Exit?"=w461:bool)
        n230 = local write "End Test"(FALSE ("End Test")) -> ()
        n231 = Select(t="UI: Front Panel State >> Close", s=w461, f="") -> (s? t:f=w458:string)
        n232 = call <vilib>:"Add State(s) to Queue__jki_lib_state_machine.vi"("State(s) in (\"\")"=w458, "State(s) at Back (\"\")"="Data: Cleanup\nExit") -> ("States Out"=w456:string)  [unwired: 13 in]
        n233 = call <vilib>:"Add State(s) to Queue__jki_lib_state_machine.vi"("State(s) in Front (\"\")"=w456, "State(s) in (\"\")"=w465) -> ("States Out"=w464:string)  [unwired: 13 in]
      }
      frame "---------- Test ----------" {
        n234 = call <vilib>:"Add State(s) to Queue__jki_lib_state_machine.vi"("State(s) in (\"\")"=w469) -> ("States Out"=w468:string)  [unwired: 14 in]
      }
      frame "Test: CheckComplete" {
        w470 = FALSE ("Blinking")
        # "If they are all finished, then exit.  \nBuild array of the number\nof draws left.\nOnly use tanks with good communcation and no temp alarm."
        n235 = call "String_in_Reference.vi"("String"=w471) -> ()  [unwired: 18 in, 1 out]
        n236 = property on="Current Draw(A)" class="DigNum (strict)"("Blinking"=w470) -> ()  [unwired: 2 in, 2 out]
        n237 = property on="Current Draw(D)" class="DigNum (strict)"("Blinking"=w470) -> ()  [unwired: 2 in, 2 out]
        n238 = property on="Current Draw(B)" class="DigNum (strict)"("Blinking"=w470) -> ()  [unwired: 2 in, 2 out]
        n239 = property on="Current Draw(C)" class="DigNum (strict)"("Blinking"=w470) -> ()  [unwired: 2 in, 2 out]
        n240 = local read "Alarm A"() -> (w483:bool)
        n241 = local read "Alarm D"() -> (w473:bool)
        n242 = local read "Alarm B"() -> (w480:bool)
        n243 = local read "Alarm C"() -> (w475:bool)
        n244 = local read "ComB"() -> (w477:bool)
        n245 = local read "ComD"() -> (w474:bool)
        n246 = local read "ComA"() -> (w482:bool)
        n247 = local read "ComC"() -> (w476:bool)
        n248 = Compound Arithmetic op=AND(w482, invert w483) -> (w481:bool)
        "result" <- w481
        n249 = Compound Arithmetic op=AND(w477, invert w480) -> (w472:bool)
        "result 2" <- w472
        n250 = Compound Arithmetic op=AND(w474, invert w473) -> (w478:bool)
        "result 4" <- w478
        n251 = Compound Arithmetic op=AND(w476, invert w475) -> (w479:bool)
        "result 3" <- w479
        n252 = case shown="True" w481 {
          tunnel: [0 w512] -> w490
          frame False {
          }
          frame True {
            n253 = Subtract(x="Num Draws (A)", y="Current Draw(A)") -> (x-y=w512:i32)
          }
        }
        n254 = case shown="True" w472 {
          tunnel: [0 w508] -> w491
          frame False {
          }
          frame True {
            n255 = Subtract(x="Num Draws (B)", y="Current Draw(B)") -> (x-y=w508:i32)
          }
        }
        n256 = case shown="True" w479 {
          tunnel: [0 w504] -> w492
          frame False {
          }
          frame True {
            n257 = Subtract(x="Num Draws (C)", y="Current Draw(C)") -> (x-y=w504:i32)
          }
        }
        n258 = case shown="True" w478 {
          tunnel: [0 w500] -> w493
          frame False {
          }
          frame True {
            n259 = Subtract(x="Num Draws (D)", y="Current Draw(D)") -> (x-y=w500:i32)
          }
        }
        n260 = Build Array(w490, w491, w492, w493) -> (w487:i32[])
        n261 = Add Array Elements(numeric array=w487) -> (sum=w485:i32)
        "Draws Left" <- w485
        n262 = To Long Integer(number=w485) -> (32bit integer=w484:i32)
        n263 = case shown="1, Default" w484 {
          tunnel: ["Exit" ("State(s) at Back (\"\")") "Test: Wait for Power Off" ("State(s) at Back (\"\")")] -> w486
          frame 0 {
          }
          frame 1, Default {
          }
        }
        n264 = Bundle By Name(cluster=w489, "DrawsLeft"=w487) -> (w488:T15)
        n265 = call <vilib>:"Add State(s) to Queue__jki_lib_state_machine.vi"("State(s) in Front (\"\")"=w486, "State(s) in (\"\")"=w496) -> ("States Out"=w495:string)  [unwired: 13 in]
      }
      frame "Test: Wait for Power Off" {
        # "Select from the tanks with no power on."
        # "Main Test Loop: Decides which Tank to Run, and starts that sequence."
        n266 = Unbundle By Name(w542) -> ("DrawsLeft"=w530:i32[], "semaphore"=w518:T4, "RLT Equipment.MW100"=w517:refnum<visa-resource-name>)
        n267 = flat-sequence {
          tunnel: w517 -> [w546]
          tunnel: [w546] -> w516
          frame #0 {
            n268 = property on="Pause test" class="Bool (strict)"("Visible"=TRUE) -> ()  [unwired: 2 in, 2 out]
          }
        }
        n269 = Greater Than 0?(x=w530) -> (x > 0?=w529:bool[])
        n270 = Index Array(array=w529, index #1=0 ("index"), index #2=1 ("index"), index #3=2 ("index"), index #4=3 ("index")) -> (element #1=w524:bool, element #2=w523:bool, element #3=w522:bool, element #4=w525:bool)
        n271 = while {
          tunnel: [w587] -> w541
          tunnel: w525 -> [w585]
          tunnel: w524 -> [w584]
          tunnel: w523 -> [w583]
          tunnel: w522 -> [w582]
          tunnel: [w568] -> w521
          tunnel: w520 -> [w566]
          tunnel: [w565] -> w519
          tunnel: w518 -> [w564]
          tunnel: w516 -> [w563]
          tunnel: [FALSE ("Visible")] -> w515
          i -> [w559]
          stop <- w556 stop-if-true
          n272 = Equal To 0?(x=w559) -> (x = 0?=w554:bool)
          n273 = case shown="True" w585 {
            tunnel: [FALSE w615] -> w589
            tunnel: w554 -> [_ w614]
            frame False {
            }
            frame True {
              n274 = local read "POWERD"() -> (w616:T5)
              n275 = call "HEWH Power Off Check.vi"("input cluster"=w616, "Init"=w614) -> ("Heat Off, Really"=w615:bool)  [unwired: 12 in, 1 out]
            }
          }
          n276 = case shown="True" w582 {
            tunnel: [FALSE w604] -> w590
            tunnel: w554 -> [_ w602]
            frame False {
            }
            frame True {
              n277 = local read "POWERC"() -> (w603:T5)
              n278 = call "HEWH Power Off Check.vi"("input cluster"=w603, "Init"=w602) -> ("Heat Off, Really"=w604:bool)  [unwired: 12 in, 1 out]
            }
          }
          n279 = case shown="True" w584 {
            tunnel: [FALSE w612] -> w592
            tunnel: w554 -> [_ w610]
            frame False {
            }
            frame True {
              n280 = local read "POWERA"() -> (w611:T5)
              n281 = call "HEWH Power Off Check.vi"("input cluster"=w611, "Init"=w610) -> ("Heat Off, Really"=w612:bool)  [unwired: 12 in, 1 out]
            }
          }
          n282 = case shown="True" w583 {
            tunnel: [FALSE w608] -> w591
            tunnel: w554 -> [_ w606]
            frame False {
            }
            frame True {
              n283 = local read "POWERB"() -> (w607:T5)
              n284 = call "HEWH Power Off Check.vi"("input cluster"=w607, "Init"=w606) -> ("Heat Off, Really"=w608:bool)  [unwired: 12 in, 1 out]
            }
          }
          n285 = Quotient & Remainder(x=w559, y="FlowPoll Rate") -> (x-y*floor(x/y)=w561:i32)  [unwired: 1 out]
          n286 = Equal To 0?(x=w561) -> (x = 0?=w562:bool)
          n287 = case shown="True" w562 {
            tunnel: w566 -> [w594 w600]
            tunnel: [w594 w599] -> w565
            tunnel: w564 -> [_ w598]
            tunnel: w563 -> [_ w597]
            frame False {
            }
            frame True {
              n288 = call "MW100_Read_GAL_Flow.vi"("MW100"=w597, "Semiphore"=w598, "Error In"=w600) -> ("Gallons"=w595:dbl, "Flow(GPM)"=w596:dbl, "Error Out"=w599:errorcluster)  [unwired: 8 in, 2 out]
              n289 = local write "Flow"(w596) -> ()
              n290 = local write "M*(Gal)"(w595) -> ()
            }
          }
          n291 = local read "Alarm A"() -> (w572:bool)
          n292 = local read "Alarm D"() -> (w578:bool)
          n293 = local read "Alarm B"() -> (w574:bool)
          n294 = local read "Alarm C"() -> (w576:bool)
          n295 = Compound Arithmetic op=OR(w592, w591, w590, w589) -> (w569:bool)
          n296 = Build Array(w592, w591, w590, w589) -> (w588:bool[])
          n297 = local read "T1 ComTimer"() -> (w593:i32)
          n298 = local read "ComB"() -> (w573:bool)
          n299 = local read "ComD"() -> (w577:bool)
          n300 = local read "ComA"() -> (w571:bool)
          n301 = local read "ComC"() -> (w575:bool)
          n302 = Boolean To (0,1)(Boolean=w588) -> (0, 1=w587:i16[])
          n303 = Compound Arithmetic op=AND(invert w574, w573) -> (w580:bool)
          n304 = Compound Arithmetic op=AND(invert w572, w571) -> (w579:bool)
          n305 = Compound Arithmetic op=AND(invert w576, w575) -> (w581:bool)
          n306 = Compound Arithmetic op=AND(invert w578, w577) -> (w570:bool)
          n307 = To Unsigned Long Integer(number=w593) -> (unsigned 32bit integer=w567:u32)
          n308 = Compound Arithmetic op=AND(invert w579, invert w580, invert w581, invert w570) -> (w568:bool)
          n309 = Compound Arithmetic op=OR(w568, w569) -> (w557:bool)
          n310 = Compound Arithmetic op=AND(w557, invert "Pause test") -> (w556:bool)
          n311 = call "String_in_Reference.vi"("String"="Waiting for Power Off") -> ()  [unwired: 18 in, 1 out]
          n312 = Wait (ms)(milliseconds to wait=w567) -> ()  [unwired: 1 out]
        }
        n313 = property on="Pause test" class="Bool (strict)"("Visible"=w515) -> ()  [unwired: 2 in, 2 out]
        n314 = case shown="False" w521 {
          tunnel: ["Test: Purge >> X\nTest: Set Direction >> X\nTest: Draw >> X\nTest: Stop Flow >> X\nTest: CheckComplete" "Exit"] -> w538
          frame False {
          }
          frame True {
            # "In case com error or alarms"
          }
        }
        n315 = Multiply(x=w530, y=w541) -> (x*y=w540:i32[])
        n316 = Array Max & Min(array=w540) -> (max value=w539:i32)  [unwired: 3 out]
        n317 = Search 1D Array(1D array=w540, element=w539) -> (index of element=w535:i32)  [unwired: 1 in]
        n318 = case shown="3" w535 {
          tunnel: ["A" ("search string") "B" ("search string") "C" ("search string") "D" ("search string")] -> w533
          frame 0, Default {
          }
          frame 1 {
          }
          frame 2 {
          }
          frame 3 {
          }
        }
        n319 = Search and Replace String(replace all?=TRUE ("replace all? (F)"), input string=w538, search string="X", replace string=w533) -> (result string=w543:string)  [unwired: 4 in, 3 out]
        n320 = Concatenate Strings("Testing Tank " ("string"), w533) -> (w532:string)
        n321 = call "String_in_Reference.vi"("String"=w532) -> ()  [unwired: 18 in, 1 out]
        n322 = call <vilib>:"Add State(s) to Queue__jki_lib_state_machine.vi"("State(s) in Front (\"\")"=w543, "State(s) in (\"\")"=w545) -> ("States Out"=w544:string)  [unwired: 13 in]
      }
      frame "Test: Set Direction" {
        n323 = case shown="\"D\"" w626 {
          tunnel: [w646 w650 w654 w658] -> w622
          tunnel: [w643 w647 w651 w655] -> w631
          tunnel: [w644 w648 w652 w656] -> w630
          frame "A", Default {
            w646 = u16 0 items=["A", "B", "C", "D"] ("Valve Bank")
            n324 = local read "Current Draw(A)"() -> (w645:i32)
            n325 = local read "FileNameA"() -> (w643:path)
            n326 = Increment(x=w645) -> (x+1=w644:i32)
            n327 = local write "Current Draw(A)"(w644) -> ()
          }
          frame "B" {
            w650 = u16 1 items=["A", "B", "C", "D"] ("Valve Bank")
            n328 = local read "Current Draw(B)"() -> (w649:i32)
            n329 = Increment(x=w649) -> (x+1=w648:i32)
            n330 = local read "FileNameB"() -> (w647:path)
            n331 = local write "Current Draw(B)"(w648) -> ()
          }
          frame "C" {
            w654 = u16 2 items=["A", "B", "C", "D"] ("Valve Bank")
            n332 = local read "Current Draw(C)"() -> (w653:i32)
            n333 = Increment(x=w653) -> (x+1=w652:i32)
            n334 = local read "FileNameC"() -> (w651:path)
            n335 = local write "Current Draw(C)"(w652) -> ()
          }
          frame "D" {
            w658 = u16 3 items=["A", "B", "C", "D"] ("Valve Bank")
            n336 = local read "Current Draw(D)"() -> (w657:i32)
            n337 = local read "FileNameD"() -> (w655:path)
            n338 = Increment(x=w657) -> (x+1=w656:i32)
            n339 = local write "Current Draw(D)"(w656) -> ()
          }
        }
        n340 = Unbundle By Name(w632) -> ("semaphore"=w621:T4, "RLT Equipment.MW100"=w623:refnum<visa-resource-name>)
        n341 = Number To Decimal String(number=w630) -> (decimal integer string=w628:string)  [unwired: 1 in]
        n342 = Concatenate Strings("Start Draw" ("String"), w628) -> (w627:string)
        n343 = call "Log String to Spreadsheet.vi"("String"=w627, "FileName"=w631) -> ()  [unwired: 9 in, 1 out]
        n344 = disable-structure shown="Enabled" {
          disable-tunnel: w625 -> [w641 w642]
          disable-tunnel: [w640 w642] -> w624
          disable-tunnel: w623 -> [w639 _]
          disable-tunnel: w621 -> [w638 _]
          frame Disabled {
            n345 = call "YKMW100 Computation Control.vi"("VISA session"=w639, "Semiphore"=w638, "Mode"=T11."Reset Computation", "error in (no error)"=w641) -> ("error out"=w640:errorcluster)  [unwired: 10 in, 1 out]
          }
          frame Enabled {
          }
        }
        n346 = local read "Expansion Tank?"() -> (w620:bool)
        n347 = call "HEWH Set Valves.vi"("VISA session"=w623, "Valve Bank"=w622, "Semiphore"=w621, "Expansion Tank?"=w620, "Valve Bank Setting"=ValveBankPositions."Draw", "Error In"=w624) -> ("Error Out"=w618:errorcluster)  [unwired: 8 in, 1 out]
        n348 = case shown="No Error" w618 {
          tunnel: ["" ("State(s) in Front (\"\")") "Test: Set Direction" ("State(s) in Front (\"\")")] -> w617
          frame No Error {
          }
          frame Error {
          }
        }
        n349 = call <vilib>:"Add State(s) to Queue__jki_lib_state_machine.vi"("State(s) in Front (\"\")"=w617, "State(s) in (\"\")"=w634) -> ("States Out"=w633:string)  [unwired: 13 in]
      }
      frame "Test: Stop Flow" {
        n350 = Unbundle By Name(w669) -> ("semaphore"=w662:T4, "RLT Equipment.MW100"=w663:refnum<visa-resource-name>)
        n351 = case shown="\"A\", Default" w666 {
          tunnel: [w673 w675 w677 w679] -> w661
          tunnel: [w672 w674 w676 w678] -> w667
          frame "A", Default {
            w673 = u16 0 items=["A", "B", "C", "D"] ("Valve Bank")
            n352 = local read "FileNameA"() -> (w672:path)
          }
          frame "B" {
            w675 = u16 1 items=["A", "B", "C", "D"] ("Valve Bank")
            n353 = local read "FileNameB"() -> (w674:path)
          }
          frame "C" {
            w677 = u16 2 items=["A", "B", "C", "D"] ("Valve Bank")
            n354 = local read "FileNameC"() -> (w676:path)
          }
          frame "D" {
            w679 = u16 3 items=["A", "B", "C", "D"] ("Valve Bank")
            n355 = local read "FileNameD"() -> (w678:path)
          }
        }
        n356 = call "Log String to Spreadsheet.vi"("String"="Stop Draw", "FileName"=w667) -> ()  [unwired: 9 in, 1 out]
        n357 = local read "Expansion Tank?"() -> (w660:bool)
        n358 = call "HEWH Set Valves.vi"("VISA session"=w663, "Valve Bank"=w661, "Semiphore"=w662, "Expansion Tank?"=w660, "Valve Bank Setting"=ValveBankPositions."Heating", "Error In"=w664) -> ("Error Out"=w665:errorcluster)  [unwired: 8 in, 1 out]
        n359 = call <vilib>:"Add State(s) to Queue__jki_lib_state_machine.vi"("State(s) in (\"\")"=w671) -> ("States Out"=w670:string)  [unwired: 14 in]
      }
      frame "Test: Purge" {
        n360 = Unbundle By Name(w704) -> ("semaphore"=w682:T4, "RLT Equipment"=w703:T3, "Degree Setting(F)"=w694:dbl, "Flow Setting(GPM)"=w693:dbl, "Temp Band"=w700:dbl)
        n361 = case shown="\"A\", Default" w680 {
          tunnel: [w726 w729 w732 w735] -> w683
          tunnel: [w724 w727 w730 w733] -> w686
          frame "A", Default {
            w726 = u16 0 items=["A", "B", "C", "D"] ("Valve Bank")
            n362 = local read "FileNameA"() -> (w724:path)
            n363 = property on="Current Draw(A)" class="DigNum (strict)"("Blinking"=TRUE) -> ()  [unwired: 2 in, 2 out]
          }
          frame "B" {
            w729 = u16 1 items=["A", "B", "C", "D"] ("Valve Bank")
            n364 = local read "FileNameB"() -> (w727:path)
            n365 = property on="Current Draw(B)" class="DigNum (strict)"("Blinking"=TRUE) -> ()  [unwired: 2 in, 2 out]
          }
          frame "C" {
            w732 = u16 2 items=["A", "B", "C", "D"] ("Valve Bank")
            n366 = local read "FileNameC"() -> (w730:path)
            n367 = property on="Current Draw(C)" class="DigNum (strict)"("Blinking"=TRUE) -> ()  [unwired: 2 in, 2 out]
          }
          frame "D" {
            w735 = u16 3 items=["A", "B", "C", "D"] ("Valve Bank")
            n368 = local read "FileNameD"() -> (w733:path)
            n369 = property on="Current Draw(D)" class="DigNum (strict)"("Blinking"=TRUE) -> ()  [unwired: 2 in, 2 out]
          }
        }
        n370 = call "String_in_Reference.vi"("String"="Purging...") -> ()  [unwired: 18 in, 1 out]
        n371 = Unbundle By Name(w703) -> ("MW100"=w684:refnum<visa-resource-name>)
        n372 = call "Log String to Spreadsheet.vi"("String"="Start Purge", "error in (no error)"=w691, "FileName"=w686) -> ("error out"=w690:errorcluster)  [unwired: 8 in]
        n373 = control-ref of="Downspout Flow Chart"() -> (w696:refnum<vi>)
        n374 = control-ref of="Downspout Temp Chart"() -> (w698:refnum<vi>)
        n375 = Bundle By Name(cluster=T13 {"COM Port"="COM9", "MW100"="MW100", "AG34970"="A-34972A", "Chamber"="WT500"} ("Equipment"), "MW100"=w684) -> (w701:T13)
        n376 = call "Purge Water Sequence SM.vi"("Degree Setting"=w694, "Equipment"=w701, "Semiphore"=w682, "Flow rate setting"=w693, "Temp Band(+/- F)"=w700, "Valve Bank"=w683, "Error In"=w690, "Flow Chart Ref"=w696, "Temp Chart Ref"=w698, "Test Condition"=TestedFlowratesScenarios."Global, Purge") -> ("Downspout Flow"=→"Downspout Flow Chart":dbl, "Downspout Temp"=→"Downspout Temp Chart":dbl, "Temp Setting Out"=→"Temp Control Sig":dbl, "Error Out"=w685:errorcluster)  [unwired: 2 out]
        n377 = case shown="No Error" w685 {
          selector: w685 -> [_ w707]
          tunnel: w684 -> [_ w711]
          tunnel: w683 -> [_ w710]
          tunnel: w682 -> [_ w709]
          tunnel: w680 -> [_ w708]
          frame No Error {
          }
          frame Error {
            n378 = disable-structure shown="Enabled" {
              disable-tunnel: w711 -> [w718 _]
              disable-tunnel: w710 -> [w715 _]
              disable-tunnel: w709 -> [w714 _]
              disable-tunnel: w708 -> [_ w723]
              disable-tunnel: w707 -> [_ w721]
              frame Disabled {
                n379 = local read "Expansion Tank?"() -> (w713:bool)
                n380 = call "Intellifaucet_Driver.vi"("VISA session"=w718, "Mode"=Intellfaucet_Mode."Stop Flow", "Semiphore"=w714) -> ("VISA session out"=w716:refnum<visa-resource-name>)  [unwired: 11 in, 1 out]
                n381 = call "HEWH Set Valves.vi"("VISA session"=w716, "Valve Bank"=w715, "Semiphore"=w714, "Expansion Tank?"=w713, "Valve Bank Setting"=ValveBankPositions."Heating") -> ()  [unwired: 9 in, 2 out]
              }
              frame Enabled {
                n382 = Unbundle By Name(w721) -> ("source"=w720:string)
                n383 = Concatenate Strings(w723, ": " ("string"), w720) -> (w719:string)
                n384 = call "String_in_Reference.vi"("String"=w719) -> ()  [unwired: 18 in, 1 out]
              }
            }
          }
        }
        n385 = call <vilib>:"Add State(s) to Queue__jki_lib_state_machine.vi"("State(s) in (\"\")"=w706) -> ("States Out"=w705:string)  [unwired: 14 in]
        n386 = call "Log String to Spreadsheet.vi"("String"="End Purge", "error in (no error)"=w685, "FileName"=w686) -> ("error out"=w688:errorcluster)  [unwired: 8 in]
      }
      frame "Test: Draw" {
        n387 = Unbundle By Name(w749) -> ("semaphore"=w744:T4, "RLT Equipment.MW100"=w745:refnum<visa-resource-name>, "Flow Setting(GPM)"=w748:dbl, "Degree Setting(F)"=w739:dbl)
        n388 = local read "Draw Amount (GAL)"() -> (w738:dbl)
        n389 = flat-sequence {
          tunnel: [Intellfaucet_Mode."Start Flow" ("Mode")] -> w743
          frame #0 {
            "Drawing" <- TRUE
          }
        }
        n390 = local read "Flow Out"() -> (w742:dbl)
        n391 = call "String_in_Reference.vi"("String"="Draw in Progress") -> ()  [unwired: 18 in, 1 out]
        n392 = call "Intellifaucet_Driver.vi"("VISA session"=w745, "Mode"=w743, "Semiphore"=w744, "Error In"=w747) -> ("Error Out"=w746:errorcluster)  [unwired: 10 in, 1 out]
        n393 = call "E-Time.vi"("error in (no error)"=w746) -> ("error out"=w750:errorcluster, "Elapsed Time (sec)"=w751:dbl)  [unwired: 8 in, 1 out]
        n394 = while {
          shift-right: [w781] -> w741
          shift-left: w750 -> [w791]
          shift-right: [w764] -> _
          shift-left: w742 -> [w772]
          tunnel: w744 -> [w769]
          tunnel: w745 -> [w771]
          tunnel: w748 -> [w770]
          tunnel: w738 -> [w790]
          tunnel: w751 -> [w789]
          shift-right: [w783] -> _
          shift-left: _ -> [w784]
          tunnel: w739 -> [w767]
          tunnel: [w762] -> w737
          i -> [w786]
          stop <- w797 stop-if-true
          (unwired) TestedFlowratesScenarios."Global, Tank" ("Test Condition")
          # "GPM Target"
          # "GPM Setting"
          # "etime for draw"
          # "start time"
          n395 = Wait (ms)(milliseconds to wait=u32 250) -> ()  [unwired: 1 out]
          n396 = call "E-Time.vi"("error in (no error)"=w791) -> ("error out"=w788:errorcluster, "Elapsed Time (sec)"=w794:dbl)  [unwired: 8 in, 1 out]
          n397 = Subtract(x=w794, y=w789) -> (x-y=w768:dbl)
          n398 = Equal To 0?(x=w786) -> (x = 0?=w787:bool)
          n399 = local read "Temp Control Sig"() -> (w766:dbl)
          n400 = call "MW100_Read_GAL_Flow.vi"("MW100"=w771, "Semiphore"=w769, "Error In"=w788) -> ("Gallons"=w785:dbl, "Flow(GPM)"=w773:dbl, "Tc_down"=w763:dbl, "Error Out"=w776:errorcluster)  [unwired: 8 in, 1 out]
          "Flow" <- w773
          n401 = case shown="False" w787 {
            tunnel: [w798 w799] -> w783
            tunnel: w785 -> [_ w799]
            tunnel: w784 -> [w798 _]
            frame False {
            }
            frame True {
            }
          }
          n402 = Subtract(x=w785, y=w783) -> (x-y=w792:dbl)
          "M*(Gal)" <- w792
          n403 = local write "Downspout Temp Chart"(w763) -> ()
          n404 = local write "Downspout Flow Chart"(w773) -> ()
          n405 = Greater Or Equal?(x=w792, y=w790) -> (x >= y?=w795:bool)
          n406 = call "HEWH Flow and Temp Adjustment.vi"("MW100"=w771, "FlowReading"=w773, "Flow In"=w772, "K(0.1)"="K(0.2)", "TempReading"=w763, "Error In"=w776, "FlowTarget"=w770, "Temp Target"=w767, "Temp In"=w766, "Semiphore"=w769, "Elapsed Time (sec)"=w768) -> ("Flow Out"=w764:dbl, "Temp Out"=w765:dbl, "Error Out"=w775:errorcluster)  [unwired: 6 in]
          "Flow Out" <- w764
          n407 = local read "Stop Test Now"() -> (w782:bool)
          n408 = local write "Temp Control Sig"(w765) -> ()
          n409 = Greater?(x=w768, y=20.0) -> (0:w777:bool)
          n410 = Equal To 0?(x=w773) -> (x = 0?=w778:bool)
          n411 = Unbundle By Name(w775) -> ("status"=w796:bool)
          n412 = And(x=w778, y=w777) -> (x .and. y?=w762:bool)
          n413 = Compound Arithmetic op=OR(w762, w796, w795, w782) -> (w797:bool)
          n414 = call "Error Bool Enumerator.vi"("Error Enum"=HEWH_Error_Enumeration."Flow = 0 During Draw after 20s", "Error In"=w775, "Error?"=w762) -> ("Error Out"=w781:errorcluster)  [unwired: 6 in]
        }
        n415 = call <vilib>:"Add State(s) to Queue__jki_lib_state_machine.vi"("State(s) in (\"\")"=w753) -> ("States Out"=w752:string)  [unwired: 14 in]
        n416 = case shown="True" w737 {
          tunnel: w736 -> [_ w754]
          frame False {
          }
          frame True {
            n417 = case shown="\"C\"" w754 {
              frame "A", Default {
                "No Draw A" <- TRUE ("Blinking")
              }
              frame "B" {
                "No Draw B" <- TRUE ("Blinking")
              }
              frame "C" {
                "No Draw C" <- TRUE ("Blinking")
              }
              frame "D" {
                "No Draw D" <- TRUE ("No Draw D")
              }
            }
          }
        }
        n418 = flat-sequence {
          tunnel: w741 -> [_]
          frame #0 {
            n419 = local write "Drawing"(FALSE) -> ()
          }
        }
      }
    }
  }
  "error out" <- w12
  "Finish" <- w1
  n420 = while {
    tunnel: w4 -> [_]
    i -> [w803]
    stop <- w805 stop-if-true
    n421 = local read "T1 ComTimer"() -> (w804:i32)
    n422 = event shown="[1] \"Stop Test Now\": Value Change" {
      selector: _ -> [_ _]
      dyn-events: _ -> [_ _]
      timeout: w804 -> [_ _]
      event Timeout {
        n423 = event-data() -> ()  [unwired: 1 in, 2 out]
        n424 = call "String_in_Reference.vi"() -> ("String Out"=w806:string)  [unwired: 19 in]
        n425 = local write "Status Message"(w806) -> ()
        n426 = call "E-Time.vi"() -> ("Elapsed Time (sec)"=w807:dbl)  [unwired: 9 in, 2 out]
        n427 = local write "Elapsed Time"(w807) -> ()
      }
      event "Stop Test Now": Value Change {
        n428 = event-data() -> ()  [unwired: 1 in, 5 out]
        n429 = local read "Save File Directory"() -> (w808:path)
        n430 = stacked-sequence {
          tunnel: w808 -> [_ w814 w827 w840 w853 _ _ _]
          tunnel: "Stopped by user." ("String") -> [_ w813 w826 w839 w852 w865 _ _]
          frame #0 {
            n431 = local read "MW100 Semiphore"() -> (w811:T4)
            n432 = call "Intellifaucet_Driver.vi"("VISA session"=refnum<visa-resource-name> "MW100", "Mode"=Intellfaucet_Mode."Stop Flow", "Semiphore"=w811) -> ()  [unwired: 11 in, 2 out]
          }
          frame #1 {
            n433 = local read "FileNameA"() -> (w816:path)
            n434 = call "Log String to Spreadsheet.vi"("String"=w813, "FileName"=w816) -> ("error out"=w815:errorcluster)  [unwired: 9 in]
            n435 = call <vilib>:"Check if File or Folder Exists.vi"("error in (no error)"=w815, "path"=w816) -> ("file or folder exists?"=w817:bool)  [unwired: 7 in, 2 out]
            n436 = case shown="True" w817 {
              tunnel: w816 -> [_ w822]
              tunnel: w814 -> [_ w818]
              frame False {
              }
              frame True {
                n437 = Strip Path(path=w822) -> (name=w821:string)  [unwired: 1 out]
                n438 = Search and Replace String(input string=w821, search string=".tmp", replace string=".csv" ("search string")) -> (result string=w820:string, error out=w825:errorcluster)  [unwired: 5 in, 2 out]
                n439 = Build Path(base path=w818, name or relative path=w820) -> (appended path=w819:path)
                n440 = Move(source path=w822, error in=w825, 10:w819) -> ()  [unwired: 2 in, 3 out]
              }
            }
          }
          frame #2 {
            n441 = local read "FileNameB"() -> (w828:path)
            n442 = call "Log String to Spreadsheet.vi"("String"=w826, "FileName"=w828) -> ("error out"=w829:errorcluster)  [unwired: 9 in]
            n443 = call <vilib>:"Check if File or Folder Exists.vi"("error in (no error)"=w829, "path"=w828) -> ("file or folder exists?"=w830:bool)  [unwired: 7 in, 2 out]
            n444 = case shown="True" w830 {
              tunnel: w828 -> [_ w835]
              tunnel: w827 -> [_ w831]
              frame False {
              }
              frame True {
                n445 = Strip Path(path=w835) -> (name=w834:string)  [unwired: 1 out]
                n446 = Search and Replace String(input string=w834, search string=".tmp", replace string=".csv" ("search string")) -> (result string=w833:string, error out=w838:errorcluster)  [unwired: 5 in, 2 out]
                n447 = Build Path(base path=w831, name or relative path=w833) -> (appended path=w832:path)
                n448 = Move(source path=w835, error in=w838, 10:w832) -> ()  [unwired: 2 in, 3 out]
              }
            }
          }
          frame #3 {
            n449 = local read "FileNameC"() -> (w841:path)
            n450 = call "Log String to Spreadsheet.vi"("String"=w839, "FileName"=w841) -> ("error out"=w842:errorcluster)  [unwired: 9 in]
            n451 = call <vilib>:"Check if File or Folder Exists.vi"("error in (no error)"=w842, "path"=w841) -> ("file or folder exists?"=w843:bool)  [unwired: 7 in, 2 out]
            n452 = case shown="True" w843 {
              tunnel: w841 -> [_ w848]
              tunnel: w840 -> [_ w844]
              frame False {
              }
              frame True {
                n453 = Strip Path(path=w848) -> (name=w847:string)  [unwired: 1 out]
                n454 = Search and Replace String(input string=w847, search string=".tmp", replace string=".csv" ("search string")) -> (result string=w846:string, error out=w851:errorcluster)  [unwired: 5 in, 2 out]
                n455 = Build Path(base path=w844, name or relative path=w846) -> (appended path=w845:path)
                n456 = Move(source path=w848, error in=w851, 10:w845) -> ()  [unwired: 2 in, 3 out]
              }
            }
          }
          frame #4 {
            n457 = local read "FileNameD"() -> (w854:path)
            n458 = call "Log String to Spreadsheet.vi"("String"=w852, "FileName"=w854) -> ("error out"=w855:errorcluster)  [unwired: 9 in]
            n459 = call <vilib>:"Check if File or Folder Exists.vi"("error in (no error)"=w855, "path"=w854) -> ("file or folder exists?"=w856:bool)  [unwired: 7 in, 2 out]
            n460 = case shown="True" w856 {
              tunnel: w854 -> [_ w861]
              tunnel: w853 -> [_ w857]
              frame False {
              }
              frame True {
                n461 = Strip Path(path=w861) -> (name=w860:string)  [unwired: 1 out]
                n462 = Search and Replace String(input string=w860, search string=".tmp", replace string=".csv" ("search string")) -> (result string=w859:string, error out=w864:errorcluster)  [unwired: 5 in, 2 out]
                n463 = Build Path(base path=w857, name or relative path=w859) -> (appended path=w858:path)
                n464 = Move(source path=w861, error in=w864, 10:w858) -> ()  [unwired: 2 in, 3 out]
              }
            }
          }
          frame #5 {
            n465 = local read "Computer Name"() -> (w866:string)
            n466 = local read "Ver."() -> (w867:string)
            n467 = property class="App"() -> ("App.Name"=w869:string)  [unwired: 2 in, 2 out]
            n468 = local read "IP Add"() -> (w870:string)
            n469 = call <vilib>:"Space Constant.vi"() -> ("String"=w868:string)
            n470 = Concatenate Strings(w870, w868, w866, w868, w869, w868, w867, w868, w865) -> (w871:string)
            n471 = call "Save Time to File.vi"("String"=w871) -> ()  [unwired: 13 in, 2 out]
          }
          frame #6 {
            n472 = global read "Global HEWH.vi" "Test Station:"() -> (w873:string)
            n473 = Concatenate Strings("robocopy c:/Data //10.2.0.10/AP2Lab/" ("command line"), w873) -> (w872:string)
            n474 = call <vilib>:"System Exec.vi"("command line"=w872) -> ()  [unwired: 7 in, 4 out]
          }
          frame #7 {
            n475 = Stop() -> ()  [unwired: 1 in]
          }
        }
      }
    }
    n476 = Quotient & Remainder(x=w803, y=2) -> (x-y*floor(x/y)=w801:i32)  [unwired: 1 out]
    n477 = Equal To 0?(x=w801) -> (x = 0?=→"UI":bool)
    n478 = local read "Finish"() -> (w805:bool)
    "UI Update Loop" <- w803
  }
  n479 = Not(x=w1) -> (.not. x?=w2:bool)
  n480 = property on="Finish" class="Bool (strict)"("Val(Sgnl)"=w1) -> ()  [unwired: 2 in, 2 out]
  n481 = local write "Start Test"(w2) -> ()
  n482 = call <vilib>:"Add State(s) to Queue__jki_lib_state_machine.vi"("State(s) in (\"\")"="Data: Initialize") -> ("States Out"=w10:string)  [unwired: 14 in]
  n483 = event shown="[0] \"Init Complete\", \"Stop Logging\": Value Change" {
    selector: _ -> [_]
    dyn-events: _ -> [_]
    timeout: _ -> [_]
    tunnel: w4 -> [_]
    event "Init Complete", "Stop Logging": Value Change {
      n484 = event-data() -> ()  [unwired: 1 in, 5 out]
      n485 = while {
        tunnel: [w952] -> w877
        i -> [w942]
        stop <- w952 stop-if-true
        n486 = local read "RLT Equipment"() -> (w950:T3)
        n487 = local read "HEWH Sample Rate"() -> (w941:i32)
        n488 = local read "Com Setting"() -> (w943:bool)
        n489 = Unbundle By Name(w950) -> ("COM B"=w947:refnum<visa-resource-name>)
        n490 = case shown="False" w943 {
          tunnel: w947 -> [w958 w963]
          tunnel: [w957 w963] -> w944
          tunnel: [w956 w961] -> w945
          tunnel: [w954 errorcluster {"status"=FALSE, "code"=0, "source"=""} ("error out")] -> w946
          tunnel: w942 -> [_ w960]
          tunnel: w941 -> [_ w959]
          frame False {
            n491 = property class="Instr"(reference=w958) -> (reference out=w957:refnum<visa-resource-name>, error out=w954:errorcluster, "Serial Settings:Number of Bytes at Serial Port"=w955:u32)  [unwired: 1 in]
            n492 = Greater Than 0?(x=w955) -> (x > 0?=w956:bool)
          }
          frame True {
            n493 = Quotient & Remainder(x=w960, y=w959) -> (x-y*floor(x/y)=w962:i32)  [unwired: 1 out]
            n494 = Equal To 0?(x=w962) -> (x = 0?=w961:bool)
          }
        }
        n495 = local read "Init Complete"() -> (w949:bool)
        n496 = And(x=w949, y=w945) -> (x .and. y?=w948:bool)
        n497 = case shown="True" w948 {
          tunnel: w944 -> [_ w966]
          tunnel: w946 -> [_ w965]
          frame False {
          }
          frame True {
            n498 = local read "Com Setting"() -> (w968:bool)
            n499 = call "HEWH RLT Gather Serial Data.vi"("Serial Port Ref"=w966, "GEA2 HyperData"=w968, "error in (no error)"=w965) -> ("Serial Data B"=w971:string[][], "error out"=w970:errorcluster)  [unwired: 11 in]
            n500 = local write "Serial Data B"(w971) -> ()
            n501 = Unbundle By Name(w970) -> ("status"=w969:bool)
            n502 = Not(x=w969) -> (.not. x?=→"ComB":bool)
          }
        }
        n503 = local read "T1 ComTimer"() -> (w953:i32)
        n504 = local read "Stop Logging"() -> (w952:bool)
        n505 = To Unsigned Long Integer(number=w953) -> (unsigned 32bit integer=w951:u32)
        n506 = Wait (ms)(milliseconds to wait=w951) -> ()  [unwired: 1 out]
      }
      "Stopped Serial B" <- w877
      n507 = while {
        tunnel: [w921] -> w876
        i -> [w911]
        stop <- w921 stop-if-true
        n508 = local read "RLT Equipment"() -> (w918:T3)
        n509 = local read "HEWH Sample Rate"() -> (w910:i32)
        n510 = local read "Com Setting"() -> (w912:bool)
        n511 = Unbundle By Name(w918) -> ("COM C"=w916:refnum<visa-resource-name>)
        n512 = case shown="True" w912 {
          tunnel: w916 -> [w927 w932]
          tunnel: [w926 w932] -> w915
          tunnel: [w925 w928] -> w913
          tunnel: [w923 errorcluster {"status"=FALSE, "code"=0, "source"=""} ("error out")] -> w914
          tunnel: w911 -> [_ w930]
          tunnel: w910 -> [_ w929]
          frame False {
            n513 = property class="Instr"(reference=w927) -> (reference out=w926:refnum<visa-resource-name>, error out=w923:errorcluster, "Serial Settings:Number of Bytes at Serial Port"=w924:u32)  [unwired: 1 in]
            n514 = Greater Than 0?(x=w924) -> (x > 0?=w925:bool)
          }
          frame True {
            n515 = Quotient & Remainder(x=w930, y=w929) -> (x-y*floor(x/y)=w931:i32)  [unwired: 1 out]
            n516 = Equal To 0?(x=w931) -> (x = 0?=w928:bool)
          }
        }
        n517 = local read "Init Complete"() -> (w919:bool)
        n518 = And(x=w919, y=w913) -> (x .and. y?=w917:bool)
        n519 = case shown="True" w917 {
          tunnel: w915 -> [_ w935]
          tunnel: w914 -> [_ w934]
          frame False {
          }
          frame True {
            n520 = local read "Com Setting"() -> (w937:bool)
            n521 = call "HEWH RLT Gather Serial Data.vi"("Serial Port Ref"=w935, "GEA2 HyperData"=w937, "error in (no error)"=w934) -> ("Serial Data B"=w940:string[][], "error out"=w939:errorcluster)  [unwired: 11 in]
            n522 = local write "Serial Data C"(w940) -> ()
            n523 = Unbundle By Name(w939) -> ("status"=w938:bool)
            n524 = Not(x=w938) -> (.not. x?=→"ComC":bool)
          }
        }
        n525 = local read "T1 ComTimer"() -> (w922:i32)
        n526 = local read "Stop Logging"() -> (w921:bool)
        n527 = To Unsigned Long Integer(number=w922) -> (unsigned 32bit integer=w920:u32)
        n528 = Wait (ms)(milliseconds to wait=w920) -> ()  [unwired: 1 out]
      }
      "Stopped Serial C" <- w876
      n529 = while {
        tunnel: [w890] -> w875
        i -> [w880]
        stop <- w890 stop-if-true
        n530 = local read "RLT Equipment"() -> (w888:T3)
        n531 = local read "HEWH Sample Rate"() -> (w879:i32)
        n532 = local read "Com Setting"() -> (w881:bool)
        n533 = Unbundle By Name(w888) -> ("COM D"=w885:refnum<visa-resource-name>)
        n534 = case shown="True" w881 {
          tunnel: w885 -> [w896 w901]
          tunnel: [w895 w901] -> w884
          tunnel: [w894 w899] -> w882
          tunnel: [w892 errorcluster {"status"=FALSE, "code"=0, "source"=""} ("error out")] -> w883
          tunnel: w880 -> [_ w898]
          tunnel: w879 -> [_ w897]
          frame False {
            n535 = property class="Instr"(reference=w896) -> (reference out=w895:refnum<visa-resource-name>, error out=w892:errorcluster, "Serial Settings:Number of Bytes at Serial Port"=w893:u32)  [unwired: 1 in]
            n536 = Greater Than 0?(x=w893) -> (x > 0?=w894:bool)
          }
          frame True {
            n537 = Quotient & Remainder(x=w898, y=w897) -> (x-y*floor(x/y)=w900:i32)  [unwired: 1 out]
            n538 = Equal To 0?(x=w900) -> (x = 0?=w899:bool)
          }
        }
        n539 = local read "Init Complete"() -> (w887:bool)
        n540 = And(x=w887, y=w882) -> (x .and. y?=w886:bool)
        n541 = case shown="True" w886 {
          tunnel: w884 -> [_ w904]
          tunnel: w883 -> [_ w903]
          frame False {
          }
          frame True {
            n542 = local read "Com Setting"() -> (w906:bool)
            n543 = call "HEWH RLT Gather Serial Data.vi"("Serial Port Ref"=w904, "GEA2 HyperData"=w906, "error in (no error)"=w903) -> ("Serial Data B"=w909:string[][], "error out"=w908:errorcluster)  [unwired: 11 in]
            n544 = local write "Serial Data D"(w909) -> ()
            n545 = Unbundle By Name(w908) -> ("status"=w907:bool)
            n546 = Not(x=w907) -> (.not. x?=→"ComD":bool)
          }
        }
        n547 = local read "T1 ComTimer"() -> (w891:i32)
        n548 = local read "Stop Logging"() -> (w890:bool)
        n549 = To Unsigned Long Integer(number=w891) -> (unsigned 32bit integer=w889:u32)
        n550 = Wait (ms)(milliseconds to wait=w889) -> ()  [unwired: 1 out]
      }
      "Stopped Serial D" <- w875
      n551 = while {
        tunnel: [w986] -> w878
        i -> [w976]
        stop <- w986 stop-if-true
        n552 = local read "Gather Data Period"() -> (w975:i32)
        n553 = local read "RLT Equipment"() -> (w984:T3)
        n554 = Divide(x=w975, y="Divisor") -> (x/y=w973:dbl)
        n555 = local read "Com Setting"() -> (w979:bool)
        n556 = To Long Integer(number=w973) -> (32bit integer=w972:i32)
        "HEWH Sample Rate" <- w972
        n557 = Unbundle By Name(w984) -> ("COM A"=w983:refnum<visa-resource-name>)
        n558 = local read "Init Complete"() -> (w987:bool)
        n559 = case shown="True" w979 {
          tunnel: w983 -> [w992 w997]
          tunnel: [w991 w997] -> w982
          tunnel: [w990 w993] -> w981
          tunnel: [w988 errorcluster {"status"=FALSE, "code"=0, "source"=""} ("error out")] -> w980
          tunnel: w976 -> [_ w996]
          tunnel: w972 -> [_ w995]
          frame False {
            n560 = property class="Instr"(reference=w992) -> (reference out=w991:refnum<visa-resource-name>, error out=w988:errorcluster, "Serial Settings:Number of Bytes at Serial Port"=w989:u32)  [unwired: 1 in]
            n561 = Greater Than 0?(x=w989) -> (x > 0?=w990:bool)
          }
          frame True {
            n562 = Quotient & Remainder(x=w996, y=w995) -> (x-y*floor(x/y)=w994:i32)  [unwired: 1 out]
            n563 = Equal To 0?(x=w994) -> (x = 0?=w993:bool)
          }
        }
        n564 = And(x=w987, y=w981) -> (x .and. y?=w985:bool)
        n565 = case shown="True" w985 {
          tunnel: w982 -> [_ w1000]
          tunnel: w980 -> [_ w999]
          frame False {
          }
          frame True {
            n566 = local read "Com Setting"() -> (w1001:bool)
            n567 = call "HEWH RLT Gather Serial Data.vi"("Serial Port Ref"=w1000, "GEA2 HyperData"=w1001, "error in (no error)"=w999) -> ("Serial Data B"=w1004:string[][], "error out"=w1003:errorcluster)  [unwired: 11 in]
            n568 = local write "Serial Data A"(w1004) -> ()
            n569 = Unbundle By Name(w1003) -> ("status"=w1002:bool)
            n570 = Not(x=w1002) -> (.not. x?=→"ComA":bool)
          }
        }
        n571 = local read "Stop Logging"() -> (w986:bool)
        n572 = local read "T1 ComTimer"() -> (w977:i32)
        n573 = To Unsigned Long Integer(number=w977) -> (unsigned 32bit integer=w978:u32)
        n574 = Wait (ms)(milliseconds to wait=w978) -> ()  [unwired: 1 out]
      }
      "Stopped Serial A" <- w878
    }
  }
  n575 = while "Data Acquisition Steps" {
    shift-right: [w1011] -> _
    shift-left: _ -> [w1010]
    shift-right: [w1014] -> _
    shift-left: _ -> [w1009]
    shift-right: [w1013] -> _
    shift-left: w10 -> [w1015]
    shift-right: [w1008] -> _
    shift-left: 0.0 ("Elapsed Time (sec)") -> [w1007]
    tunnel: w4 -> [_]
    stop <- w1012 stop-if-true
    n576 = call <vilib>:"Parse State Queue__jki_lib_state_machine.vi"("State Queue"=w1015, "Error In (no error)"=w1009) -> ("Remaining States"=w1017:string, "Current State"=w1018:string, "Arguments"=w1016:string)  [unwired: 11 in]
    n577 = case shown="\"Data: Queue\"" w1018 {
      selector: w1018 -> [_ w1062 _ _ _ _ _ _ _ _]
      tunnel: w1017 -> [w1029 w1066 w1079 w1086 w1105 w1115 w1133 w1143 w1154 w1172]
      tunnel: w1016 -> [_ _ _ _ _ _ _ _ _ _]
      tunnel: w1010 -> [w1027 w1064 w1076 w1084 w1102 _ w1125 w1141 w1144 w1169]
      tunnel: [w1026 w1068 errorcluster {"status"=FALSE, "code"=0, "source"=""} ("error out") w1081 w1103 w1113 w1130 w1139 w1147 w1170] -> w1014
      tunnel: w1009 -> [w1025 w1067 w1075 w1082 w1103 w1113 w1131 w1139 w1148 w1170]
      tunnel: [w1028 w1065 w1078 w1085 w1104 w1114 w1132 w1142 w1153 w1171] -> w1013
      tunnel: [_ _ _ w1083 _ _ _ _ _ _] -> w1012
      tunnel: [w1024 w1064 w1076 w1084 w1102 w1112 w1124 w1140 w1152 w1169] -> w1011
      tunnel: "Gather Data Period" -> [w1023 _ _ _ _ _ _ _ _ _]
      tunnel: [w1021 w1061 w1073 w1080 w1101 w1110 w1123 w1134 w1145 w1165] -> w1008
      tunnel: w1007 -> [w1020 w1061 w1073 w1080 w1101 w1110 w1123 w1134 w1145 w1165]
      frame "", "Idle" {
        n578 = call "E-Time.vi"() -> ("Elapsed Time (sec)"=w1019:dbl)  [unwired: 9 in, 2 out]
        n579 = call "RLT Timeout Calc.vi"("Complete time"=w1019, "Gather Data Period"=w1023, "Start Time"=w1020) -> ("coerced(x)"=w1022:i32)  [unwired: 8 in]
        n580 = event shown="[0] Timeout" {
          selector: _ -> [_ _]
          dyn-events: _ -> [_ _]
          timeout: w1022 -> [_ _]
          tunnel: w1029 -> [w1036 w1060]
          tunnel: [w1035 w1059] -> w1028
          tunnel: w1027 -> [w1033 w1057]
          tunnel: [w1034 w1058] -> w1026
          tunnel: w1025 -> [w1034 w1058]
          tunnel: [w1033 w1057] -> w1024
          tunnel: [w1030 _] -> w1021
          event Timeout {
            n581 = local read "Init Complete"() -> (w1032:bool)
            n582 = event-data() -> ()  [unwired: 1 in, 1 out]
            n583 = call "E-Time.vi"() -> ("Elapsed Time (sec)"=w1030:dbl)  [unwired: 9 in, 2 out]
            n584 = case shown="True" w1032 {
              tunnel: [w1038 w1042] -> w1031
              tunnel: w1030 -> [_ _]
              frame False {
                n585 = local read "Finish"() -> (w1037:bool)
                n586 = case shown="False" w1037 {
                  tunnel: ["" "Exit"] -> w1038
                  frame False {
                  }
                  frame True {
                  }
                }
              }
              frame True {
                n587 = local read "Finish"() -> (w1041:bool)
                n588 = case shown="False" w1041 {
                  tunnel: ["Data: Acquire 1\nData: Acquire 2\nData: Acquire 3\nData: Queue" "Exit"] -> w1042
                  frame False {
                    w1045 = 5  # Q Limit
                    # "Wait for Q to empty."
                    n589 = local read "DataQ"() -> (w1047:refnum<queue>)
                    n590 = Get Queue Status(queue=w1047) -> (queue out=w1043:refnum<queue>, # elements in queue=w1046:i32)  [unwired: 2 in, 6 out]
                    n591 = Greater Or Equal?(x=w1046, y=w1045) -> (x >= y?=w1044:bool)
                    n592 = case shown="True" w1044 {
                      tunnel: w1043 -> [_ w1049]
                      frame False {
                      }
                      frame True {
                        n593 = while {
                          tunnel: w1049 -> [w1053]
                          stop <- w1052 continue-if-true
                          n594 = Get Queue Status(queue=w1053) -> (# elements in queue=w1050:i32)  [unwired: 2 in, 7 out]
                          n595 = Greater Than 0?(x=w1050) -> (x > 0?=w1052:bool)
                          n596 = property on="# elements in queue" class="DigNum (strict)"("Val(Sgnl)"=w1050) -> ()  [unwired: 2 in, 2 out]
                          n597 = Wait Until Next ms Multiple(millisecond multiple=u32 150) -> ()  [unwired: 1 out]
                        }
                      }
                    }
                  }
                  frame True {
                  }
                }
              }
            }
            n598 = call <vilib>:"Add State(s) to Queue__jki_lib_state_machine.vi"("State(s) in Front (\"\")"=w1031, "State(s) in (\"\")"=w1036) -> ("States Out"=w1035:string)  [unwired: 13 in]
          }
          event Panel Close? {
            # "Discard the event because we'll close the front panel ourselves in Macro: Exit"
            # "Close Panel button (pressed) Event\n(this executes Macro: Exit to terminate the VI)"
            n599 = event-data() -> ()  [unwired: 1 in, 1 out]
            n600 = event-data("Discard?"=TRUE) -> ()  [unwired: 1 in, 1 out]
            n601 = call <vilib>:"Add State(s) to Queue__jki_lib_state_machine.vi"("State(s) in Front (\"\")"="Macro: Exit", "State(s) in (\"\")"=w1060) -> ("States Out"=w1059:string)  [unwired: 13 in]
          }
        }
      }
      frame Default {
        w1071 = 42 items=["No error", "Argument error", "Memory is full", "Out of zone", "End of file", "File already open", "Generic file I/O error", "File not found", "File permission error", "Disk is full", "Duplicate path", "Too many files open", "System feature not enabled", "Resource file not found", "Cannot add resource", "Resource not found", "Image not found", "Image memory error", "Pen does not exist", "Config type invalid", "Config token not found", "Config parse error", "Config memory error", "Bad external code format", "Bad external code offset", "External code not present", "Null window", "Destroy window error", "Null menu", "Print aborted", "Bad print record", "Print driver error", "Windows error during printing", "Memory error during printing", "Print dialog error", "Generic print error", "Invalid device refnum", "Device not found", "Device parameter error", "Device unit error", "Cannot open device", "Device call aborted", "Generic error", "Cancelled by user", "Object ID too low", "Object ID too high", "Object not in heap", "Unknown heap", "Unknown object (invalid DefProc)", "Unknown object (DefProc not in table)", "Message out of range", "Invalid (null) method", "Unknown message", "Manager call not supported", "Bad address", "Network operation in progress", "Network operation timed out", "Connection is busy", "Network attribute not supported", "Network error", "Address in use", "System out of memory", "Connection aborted", "Connection refused", "Not connected", "Already connected", "Connection closed", "Initialization error (interapplication manager)", "Bad occurrence", "Wait on unbound occurrence handler", "Occurrence queue overflow", "Datalog type conflict", "Unused", "Unrecognized type (interapplication manager)", "Memory corrupt", "Failed to make temporary DLL", "Old CIN version", "Drag socket not found", "Failed to load drop-object", "Failed to register OLE object", "Failed to release OLE object", "Format specifier type mismatch", "Unknown format specifier", "Too few format specifiers", "Too many format specifiers", "Scan failed", "Newer CIN version", "Error converting to variant", "Runtime menu error", "Password tampered", "Variant attribute not found", "Incompatible variant data type", "Event data is not available", "Event Store is not present", "Occurrence is not found", "Event Queue is not created", "Event info is not available", "Refnum passed is NULL", "Error retrieving Class GUID", "Error retrieving CoClass GUID", "Error retrieving TypeLib GUID.", "Bad built application magic bytes.", "Specific driver is different from the specific driver associated with the Logical Name.", "There is no session opened to the class driver.", "Max Error", "MAX - Error with config objects", "MAX - Error loading configuration", "MAX - Group not supported"]
        # "Current State"
        # "Do not delete, rename, or modify this frame.\n(this is used to capture unhandled states and typos)"
        # "Handle mistyped state name (developer tool)"
        n602 = Format Into String(format string="Software Exception: Unhandled State \"%s\"." ("message"), error in=w1067, w1062) -> (resulting string=w1070:string, error out=w1069:errorcluster)  [unwired: 1 in]
        n603 = call <vilib>:"Error Cluster From Error Code.vi"("show call chain? (False)"=TRUE, "error in (no error)"=w1069, "error message (\"\")"=w1070, "error code (0)"=w1071) -> ("error out"=w1068:errorcluster)  [unwired: 5 in]
        n604 = call <vilib>:"Add State(s) to Queue__jki_lib_state_machine.vi"("State(s) in (\"\")"=w1066) -> ("States Out"=w1065:string)  [unwired: 14 in]
      }
      frame "Error Handler" {
        # "Unhandled Error -- Display it"
        # "Handle any errors here.\nYou can also output any states to clean-up after errors occur"
        # "Clear error"
        n605 = call <vilib>:"General Error Handler.vi"("error in (no error)"=w1075) -> ()  [unwired: 10 in, 5 out]
        n606 = call <vilib>:"Add State(s) to Queue__jki_lib_state_machine.vi"("State(s) in Front (\"\")"="/* Post Error States", "State(s) in (\"\")"=w1079) -> ("States Out"=w1078:string)  [unwired: 13 in]
      }
      frame "Exit" {
        n607 = while {
          tunnel: [w1087] -> w1083
          tunnel: w1082 -> [w1095]
          tunnel: [w1094] -> w1081
          stop <- w1089 stop-if-true
          w1087 = TRUE
          n608 = local read "Stopped Serial A"() -> (w1090:bool)
          n609 = local read "Stopped Serial B"() -> (w1091:bool)
          n610 = local read "Stopped Serial C"() -> (w1092:bool)
          n611 = local read "Stopped Serial D"() -> (w1093:bool)
          n612 = Compound Arithmetic op=AND(w1090, w1091, w1092, w1093) -> (w1089:bool)
          n613 = case shown="True" w1089 {
            tunnel: w1095 -> [w1096 w1098]
            tunnel: [w1096 w1097] -> w1094
            frame False {
            }
            frame True {
              n614 = local read "MW100 Semiphore"() -> (w1100:T4)
              n615 = local read "Local?"() -> (w1099:bool)
              n616 = call "Semiphore-Destroy-Local.vi"("Semiphore"=w1100, "Local?"=w1099, "error in (no error)"=w1098) -> ("error out"=w1097:errorcluster)  [unwired: 16 in]
            }
          }
          n617 = property on="Stop Logging" class="Bool (strict)"("Val(Sgnl)"=w1087) -> ()  [unwired: 2 in, 2 out]
          n618 = Wait (ms)(milliseconds to wait=u32 125) -> ()  [unwired: 1 out]
          "Stop Logging" <- w1087
        }
        n619 = call <vilib>:"Add State(s) to Queue__jki_lib_state_machine.vi"("State(s) in (\"\")"=w1086) -> ("States Out"=w1085:string)  [unwired: 14 in]
      }
      frame "---------- Data ----------" {
        # "Do not put any code in this frame.\n(It is a separator no-op. You can make a copy of this frame to create a new Data frame)"
        n620 = call <vilib>:"Add State(s) to Queue__jki_lib_state_machine.vi"("State(s) in (\"\")"=w1105) -> ("States Out"=w1104:string)  [unwired: 14 in]
      }
      frame "Data: Initialize" {
        w1108 = dbl[] [] ("MW100 Data")
        w1109 = string[][] [] ("Serial Data A")
        n621 = while {
          tunnel: [w1118] -> w1106
          stop <- w1119 stop-if-true
          n622 = local read "T1 ComTimer"() -> (w1121:i32)
          n623 = To Unsigned Long Integer(number=w1121) -> (unsigned 32bit integer=w1122:u32)
          n624 = Wait (ms)(milliseconds to wait=w1122) -> ()  [unwired: 1 out]
          n625 = local read "Init Complete"() -> (w1120:bool)
          n626 = local read "Finish"() -> (w1118:bool)
          n627 = Or(x=w1120, y=w1118) -> (x .or. y?=w1119:bool)
        }
        n628 = case shown="True" w1106 {
          tunnel: ["Data: Acquire 1\nData: Acquire 2\nData: Acquire 3\nData: Queue" "Exit"] -> w1107
          frame False {
          }
          frame True {
          }
        }
        n629 = Bundle("MW100 Data"=w1108, "Serial Data A"=w1109, "Serial Data A"=w1109, "Serial Data A"=w1109, "Serial Data A"=w1109, "MW100 Data"=w1108) -> (w1112:T19)  [unwired: 1 in]
        n630 = Obtain Queue(element data type=w1112) -> (queue out=→"DataQ":refnum<queue>)  [unwired: 4 in, 2 out]
        n631 = call <vilib>:"Add State(s) to Queue__jki_lib_state_machine.vi"("State(s) in Front (\"\")"=w1107, "State(s) in (\"\")"=w1115) -> ("States Out"=w1114:string)  [unwired: 13 in]
        "MW100 Data" <- w1108
        "Serial Data A" <- w1109
        "Agilent Output Data" <- w1108
        "Serial Data B" <- w1109
        "Serial Data C" <- w1109
        "Serial Data D" <- w1109
      }
      frame "Data: Acquire 1" {
        # "Acquire MW100 Data"
        # "Gathers All data from MW100"
        n632 = local read "RLT Equipment"() -> (w1128:T3)
        n633 = local read "MW100 Semiphore"() -> (w1129:T4)
        n634 = Unbundle By Name(w1128) -> ("MW100"=w1127:refnum<visa-resource-name>)
        n635 = call "HEWH Read All MW100 Inputs.vi"("MW100"=w1127, "Semiphore"=w1129, "Error In"=w1131) -> ("All Data"=w1126:dbl[], "error out"=w1130:errorcluster)  [unwired: 10 in, 1 out]
        n636 = local write "MW100 Data"(w1126) -> ()
        n637 = Bundle By Name(cluster=w1125, "MW100 Data"=w1126) -> (w1124:T19)
        n638 = call <vilib>:"Add State(s) to Queue__jki_lib_state_machine.vi"("State(s) in (\"\")"=w1133) -> ("States Out"=w1132:string)  [unwired: 14 in]
      }
      frame "Data: Acquire 2" {
        # "Take in serial data."
        n639 = local read "Serial Data D"() -> (w1135:string[][])
        n640 = local read "Serial Data C"() -> (w1136:string[][])
        n641 = local read "Serial Data A"() -> (w1138:string[][])
        n642 = local read "Serial Data B"() -> (w1137:string[][])
        n643 = Bundle By Name(cluster=w1141, "Serial Data A"=w1138, "Serial Data A"=w1137, "Serial Data A"=w1136, "Serial Data A"=w1135) -> (w1140:T19)
        n644 = call <vilib>:"Add State(s) to Queue__jki_lib_state_machine.vi"("State(s) in (\"\")"=w1143) -> ("States Out"=w1142:string)  [unwired: 14 in]
      }
      frame "Data: Acquire 3" {
        # "Acquire Agilent Data"
        n645 = local read "Agilent Scan List"() -> (w1149:string)
        n646 = String Length(string=w1149) -> (length=w1151:i32)
        n647 = Greater Than 0?(x=w1151) -> (x > 0?=w1146:bool)
        n648 = case shown="True" w1146 {
          tunnel: [dbl[] [] ("Output Data Permutation") w1160] -> w1150
          tunnel: w1149 -> [_ w1159]
          tunnel: w1148 -> [w1156 w1158]
          tunnel: [w1156 w1157] -> w1147
          frame False {
          }
          frame True {
            n649 = local read "RLT Equipment"() -> (w1163:T3)
            n650 = Unbundle By Name(w1163) -> ("AG34970"=w1162:refnum<visa-resource-name>)
            n651 = call "Agilent Scan EZ Temperature.vi"("VISA Resource Name"=w1162, "Control"=enum16{"Initialize", "Read", "Experiment"}."Read", "error in (no error)"=w1158) -> ("Output Array"=w1164:dbl[], "error out"=w1157:errorcluster)  [unwired: 9 in, 2 out]
            n652 = call "Agilent_ScanList_Permutation.vi"("Input Data Array"=w1164, "Agilent Scan List"=w1159) -> ("Output Data Permutation"=w1160:dbl[])  [unwired: 9 in]
          }
        }
        n653 = Bundle By Name(cluster=w1144, "MW100 Data"=w1150) -> (w1152:T19)
        n654 = local write "Agilent Output Data"(w1150) -> ()
        n655 = call <vilib>:"Add State(s) to Queue__jki_lib_state_machine.vi"("State(s) in (\"\")"=w1154) -> ("States Out"=w1153:string)  [unwired: 14 in]
      }
      frame "Data: Queue" {
        # "Put Data in Queue to be used by parsing/saving code ->"
        n656 = local read "DataQ"() -> (w1168:refnum<queue>)
        n657 = Enqueue Element(queue=w1168, element=w1169) -> (queue out=w1167:refnum<queue>)  [unwired: 2 in, 2 out]
        n658 = Get Queue Status(queue=w1167) -> (# elements in queue=w1166:i32)  [unwired: 2 in, 7 out]
        "# elements in queue" <- w1166
        n659 = property on="# elements in queue" class="DigNum (strict)"("Val(Sgnl)"=w1166) -> ()  [unwired: 2 in, 2 out]
        n660 = call <vilib>:"Add State(s) to Queue__jki_lib_state_machine.vi"("State(s) in (\"\")"=w1172) -> ("States Out"=w1171:string)  [unwired: 14 in]
      }
    }
  }
  n661 = call <vilib>:"Add State(s) to Queue__jki_lib_state_machine.vi"("State(s) in (\"\")"="Data: Initialize\nUI: Initialize") -> ("States Out"=w9:string)  [unwired: 14 in]
  n662 = while "Data Procressing, Storage, Display" {
    shift-right: [w1176] -> _
    shift-left: _ -> [w1175]
    shift-right: [w1179] -> _
    shift-left: _ -> [w1173]
    shift-right: [w1178] -> _
    shift-left: w9 -> [w1180]
    tunnel: w4 -> [_]
    stop <- w1177 stop-if-true
    n663 = call <vilib>:"Parse State Queue__jki_lib_state_machine.vi"("State Queue"=w1180, "Error In (no error)"=w1173) -> ("Remaining States"=w1182:string, "Current State"=w1183:string, "Arguments"=w1181:string)  [unwired: 11 in]
    n664 = case shown="\"UI: Update\"" w1183 {
      selector: w1183 -> [_ w1210 _ _ _ _ _ _ _ _ _ _ _ _ _ _ _]
      tunnel: w1182 -> [w1190 w1214 w1226 w1231 w1297 w1303 w1371 w1393 w1408 w1414 w1424 w1454 w1499 w1553 w1603 w1629 w1653]
      tunnel: w1181 -> [_ _ _ _ _ _ _ _ _ _ _ _ _ _ _ _ _]
      tunnel: w1175 -> [w1188 w1212 w1223 w1229 w1294 w1300 w1323 w1390 w1405 w1411 w1421 w1439 w1495 w1550 w1600 w1612 w1650]
      tunnel: [w1187 w1216 errorcluster {"status"=FALSE, "code"=0, "source"=""} ("error out") w1227 w1295 w1301 w1369 w1391 w1406 w1412 w1422 w1452 w1497 w1551 w1601 w1627 w1651] -> w1179
      tunnel: w1173 -> [w1186 w1215 w1222 w1227 w1295 w1301 w1369 w1391 w1406 w1412 w1422 w1452 w1497 w1551 w1601 w1627 w1651]
      tunnel: [w1189 w1213 w1225 w1230 w1296 w1302 w1370 w1392 w1407 w1413 w1423 w1453 w1498 w1552 w1602 w1628 w1652] -> w1178
      tunnel: [_ _ _ TRUE _ _ _ _ _ _ _ _ _ _ _ _ _] -> w1177
      tunnel: [w1185 w1212 w1223 w1229 w1294 w1300 w1323 w1390 w1404 w1410 w1421 w1438 w1494 w1550 w1599 w1625 w1650] -> w1176
      tunnel: -1 ("Gather Data Period 2") -> [w1184 _ _ _ _ _ _ _ _ _ _ _ _ _ _ _ _]
      frame "", "Idle" {
        # "executes when the state queue is empty"
        n665 = event shown="[1] \"# elements in queue\": Value Change" {
          selector: _ -> [_ _ _ _]
          dyn-events: _ -> [_ _ _ _]
          timeout: w1184 -> [_ _ _ _]
          tunnel: w1190 -> [w1195 _ _ w1209]
          tunnel: [w1194 w1198 w1202 w1208] -> w1189
          tunnel: w1188 -> [w1192 w1199 w1203 w1206]
          tunnel: [w1193 w1196 w1200 w1207] -> w1187
          tunnel: w1186 -> [w1193 w1196 w1200 w1207]
          tunnel: [w1192 w1199 w1203 w1206] -> w1185
          event Timeout {
            n666 = event-data() -> ()  [unwired: 1 in, 1 out]
            n667 = call <vilib>:"Add State(s) to Queue__jki_lib_state_machine.vi"("State(s) in Front (\"\")"="Exit", "State(s) in (\"\")"=w1195) -> ("States Out"=w1194:string)  [unwired: 13 in]
          }
          event "# elements in queue": Value Change {
            n668 = event-data() -> ()  [unwired: 1 in, 6 out]
            n669 = call <vilib>:"Add State(s) to Queue__jki_lib_state_machine.vi"("State(s) in Front (\"\")"="Data: DeQueue\nData: Process\nData: Save\nUI: Update" ("State(s) in Front (\"\")")) -> ("States Out"=w1198:string)  [unwired: 14 in]
          }
          event "Finish": Value Change {
            n670 = event-data() -> ()  [unwired: 1 in, 6 out]
            n671 = call <vilib>:"Add State(s) to Queue__jki_lib_state_machine.vi"("State(s) in Front (\"\")"="Exit" ("State(s) in Front (\"\")")) -> ("States Out"=w1202:string)  [unwired: 14 in]
          }
          event Panel Close? {
            # "Discard the event because we'll close the front panel ourselves in Macro: Exit"
            # "Close Panel button (pressed) Event\n(this executes Macro: Exit to terminate the VI)"
            n672 = event-data() -> ()  [unwired: 1 in, 1 out]
            n673 = event-data("Discard?"=TRUE) -> ()  [unwired: 1 in, 1 out]
            n674 = call <vilib>:"Add State(s) to Queue__jki_lib_state_machine.vi"("State(s) in Front (\"\")"="Macro: Exit", "State(s) in (\"\")"=w1209) -> ("States Out"=w1208:string)  [unwired: 13 in]
          }
        }
      }
      frame Default {
        w1219 = 42 items=["No error", "Argument error", "Memory is full", "Out of zone", "End of file", "File already open", "Generic file I/O error", "File not found", "File permission error", "Disk is full", "Duplicate path", "Too many files open", "System feature not enabled", "Resource file not found", "Cannot add resource", "Resource not found", "Image not found", "Image memory error", "Pen does not exist", "Config type invalid", "Config token not found", "Config parse error", "Config memory error", "Bad external code format", "Bad external code offset", "External code not present", "Null window", "Destroy window error", "Null menu", "Print aborted", "Bad print record", "Print driver error", "Windows error during printing", "Memory error during printing", "Print dialog error", "Generic print error", "Invalid device refnum", "Device not found", "Device parameter error", "Device unit error", "Cannot open device", "Device call aborted", "Generic error", "Cancelled by user", "Object ID too low", "Object ID too high", "Object not in heap", "Unknown heap", "Unknown object (invalid DefProc)", "Unknown object (DefProc not in table)", "Message out of range", "Invalid (null) method", "Unknown message", "Manager call not supported", "Bad address", "Network operation in progress", "Network operation timed out", "Connection is busy", "Network attribute not supported", "Network error", "Address in use", "System out of memory", "Connection aborted", "Connection refused", "Not connected", "Already connected", "Connection closed", "Initialization error (interapplication manager)", "Bad occurrence", "Wait on unbound occurrence handler", "Occurrence queue overflow", "Datalog type conflict", "Unused", "Unrecognized type (interapplication manager)", "Memory corrupt", "Failed to make temporary DLL", "Old CIN version", "Drag socket not found", "Failed to load drop-object", "Failed to register OLE object", "Failed to release OLE object", "Format specifier type mismatch", "Unknown format specifier", "Too few format specifiers", "Too many format specifiers", "Scan failed", "Newer CIN version", "Error converting to variant", "Runtime menu error", "Password tampered", "Variant attribute not found", "Incompatible variant data type", "Event data is not available", "Event Store is not present", "Occurrence is not found", "Event Queue is not created", "Event info is not available", "Refnum passed is NULL", "Error retrieving Class GUID", "Error retrieving CoClass GUID", "Error retrieving TypeLib GUID.", "Bad built application magic bytes.", "Specific driver is different from the specific driver associated with the Logical Name.", "There is no session opened to the class driver.", "Max Error", "MAX - Error with config objects", "MAX - Error loading configuration", "MAX - Group not supported"]
        # "Current State"
        # "Do not delete, rename, or modify this frame.\n(this is used to capture unhandled states and typos)"
        # "Handle mistyped state name (developer tool)"
        n675 = Format Into String(format string="Software Exception: Unhandled State \"%s\"." ("message"), error in=w1215, w1210) -> (resulting string=w1218:string, error out=w1217:errorcluster)  [unwired: 1 in]
        n676 = call <vilib>:"Error Cluster From Error Code.vi"("show call chain? (False)"=TRUE, "error in (no error)"=w1217, "error message (\"\")"=w1218, "error code (0)"=w1219) -> ("error out"=w1216:errorcluster)  [unwired: 5 in]
        n677 = call <vilib>:"Add State(s) to Queue__jki_lib_state_machine.vi"("State(s) in (\"\")"=w1214) -> ("States Out"=w1213:string)  [unwired: 14 in]
      }
      frame "Error Handler" {
        # "Unhandled Error -- Display it"
        # "Handle any errors here.\nYou can also output any states to clean-up after errors occur"
        # "Clear error"
        n678 = call <vilib>:"General Error Handler.vi"("error in (no error)"=w1222) -> ()  [unwired: 10 in, 5 out]
        n679 = call <vilib>:"Add State(s) to Queue__jki_lib_state_machine.vi"("State(s) in Front (\"\")"="/* Post Error States", "State(s) in (\"\")"=w1226) -> ("States Out"=w1225:string)  [unwired: 13 in]
      }
      frame "Exit" {
        # "Do not put any code in this frame.\n(No errors that occur here will be handled.)"
        n680 = stacked-sequence {
          tunnel: w1227 -> [w1235 w1248 w1261 w1274 _ _]
          frame #0 {
            n681 = local read "FileNameA"() -> (w1233:path)
            n682 = call "Log String to Spreadsheet.vi"("String"="Stopped", "error in (no error)"=w1235, "FileName"=w1233) -> ("error out"=w1232:errorcluster)  [unwired: 8 in]
            n683 = call <vilib>:"Check if File or Folder Exists.vi"("error in (no error)"=w1232, "path"=w1233) -> ("file or folder exists?"=w1234:bool)  [unwired: 7 in, 2 out]
            n684 = case shown="True" w1234 {
              tunnel: w1233 -> [_ w1241]
              frame False {
              }
              frame True {
                n685 = Strip Path(path=w1241) -> (name=w1240:string)  [unwired: 1 out]
                n686 = Search and Replace String(input string=w1240, search string=".tmp", replace string=".csv" ("search string")) -> (result string=w1238:string, error out=w1244:errorcluster)  [unwired: 5 in, 2 out]
                n687 = Build Path(base path="Save File Directory", name or relative path=w1238) -> (appended path=w1237:path)
                n688 = Move(source path=w1241, error in=w1244, 10:w1237) -> ()  [unwired: 2 in, 3 out]
              }
            }
          }
          frame #1 {
            n689 = local read "FileNameB"() -> (w1245:path)
            n690 = call "Log String to Spreadsheet.vi"("String"="Stopped", "error in (no error)"=w1248, "FileName"=w1245) -> ("error out"=w1246:errorcluster)  [unwired: 8 in]
            n691 = call <vilib>:"Check if File or Folder Exists.vi"("error in (no error)"=w1246, "path"=w1245) -> ("file or folder exists?"=w1247:bool)  [unwired: 7 in, 2 out]
            n692 = case shown="True" w1247 {
              tunnel: w1245 -> [_ w1254]
              frame False {
              }
              frame True {
                n693 = Strip Path(path=w1254) -> (name=w1253:string)  [unwired: 1 out]
                n694 = local read "Save File Directory"() -> (w1250:path)
                n695 = Search and Replace String(input string=w1253, search string=".tmp", replace string=".csv" ("search string")) -> (result string=w1252:string, error out=w1257:errorcluster)  [unwired: 5 in, 2 out]
                n696 = Build Path(base path=w1250, name or relative path=w1252) -> (appended path=w1251:path)
                n697 = Move(source path=w1254, error in=w1257, 10:w1251) -> ()  [unwired: 2 in, 3 out]
              }
            }
          }
          frame #2 {
            n698 = local read "FileNameC"() -> (w1258:path)
            n699 = call "Log String to Spreadsheet.vi"("String"="Stopped", "error in (no error)"=w1261, "FileName"=w1258) -> ("error out"=w1259:errorcluster)  [unwired: 8 in]
            n700 = call <vilib>:"Check if File or Folder Exists.vi"("error in (no error)"=w1259, "path"=w1258) -> ("file or folder exists?"=w1260:bool)  [unwired: 7 in, 2 out]
            n701 = case shown="True" w1260 {
              tunnel: w1258 -> [_ w1267]
              frame False {
              }
              frame True {
                n702 = Strip Path(path=w1267) -> (name=w1266:string)  [unwired: 1 out]
                n703 = local read "Save File Directory"() -> (w1263:path)
                n704 = Search and Replace String(input string=w1266, search string=".tmp", replace string=".csv" ("search string")) -> (result string=w1265:string, error out=w1270:errorcluster)  [unwired: 5 in, 2 out]
                n705 = Build Path(base path=w1263, name or relative path=w1265) -> (appended path=w1264:path)
                n706 = Move(source path=w1267, error in=w1270, 10:w1264) -> ()  [unwired: 2 in, 3 out]
              }
            }
          }
          frame #3 {
            n707 = local read "FileNameD"() -> (w1271:path)
            n708 = call "Log String to Spreadsheet.vi"("String"="Stopped", "error in (no error)"=w1274, "FileName"=w1271) -> ("error out"=w1272:errorcluster)  [unwired: 8 in]
            n709 = call <vilib>:"Check if File or Folder Exists.vi"("error in (no error)"=w1272, "path"=w1271) -> ("file or folder exists?"=w1273:bool)  [unwired: 7 in, 2 out]
            n710 = case shown="True" w1273 {
              tunnel: w1271 -> [_ w1280]
              frame False {
              }
              frame True {
                n711 = Strip Path(path=w1280) -> (name=w1279:string)  [unwired: 1 out]
                n712 = local read "Save File Directory"() -> (w1276:path)
                n713 = Search and Replace String(input string=w1279, search string=".tmp", replace string=".csv" ("search string")) -> (result string=w1278:string, error out=w1283:errorcluster)  [unwired: 5 in, 2 out]
                n714 = Build Path(base path=w1276, name or relative path=w1278) -> (appended path=w1277:path)
                n715 = Move(source path=w1280, error in=w1283, 10:w1277) -> ()  [unwired: 2 in, 3 out]
              }
            }
          }
          frame #4 {
            n716 = local read "Computer Name"() -> (w1284:string)
            n717 = local read "Ver."() -> (w1285:string)
            n718 = property class="App"() -> ("App.Name"=w1288:string)  [unwired: 2 in, 2 out]
            n719 = local read "IP Add"() -> (w1289:string)
            n720 = call <vilib>:"Space Constant.vi"() -> ("String"=w1287:string)
            n721 = Concatenate Strings(w1289, w1287, w1284, w1287, w1288, w1287, w1285, w1287, "Comleted." ("string")) -> (w1290:string)
            n722 = call "Save Time to File.vi"("String"=w1290) -> ()  [unwired: 13 in, 2 out]
          }
          frame #5 {
            n723 = global read "Global HEWH.vi" "Test Station:"() -> (w1292:string)
            n724 = Concatenate Strings("robocopy c:/Data //10.2.0.10/AP2Lab/" ("command line"), w1292) -> (w1291:string)
            n725 = call <vilib>:"System Exec.vi"("command line"=w1291) -> ()  [unwired: 7 in, 4 out]
          }
        }
        n726 = call <vilib>:"Add State(s) to Queue__jki_lib_state_machine.vi"("State(s) in (\"\")"=w1231) -> ("States Out"=w1230:string)  [unwired: 14 in]
      }
      frame "---------- UI ----------" {
        # "Do not put any code in this frame.\n(It is a separator no-op. You can make a copy of this frame to create a new Data frame)"
        n727 = call <vilib>:"Add State(s) to Queue__jki_lib_state_machine.vi"("State(s) in (\"\")"=w1297) -> ("States Out"=w1296:string)  [unwired: 14 in]
      }
      frame "UI: Initialize" {
        w1298 = u32 6618880 ("Color Box")
        w1299 = T5 {"UE"=TRUE, "LE"=TRUE, "COMP"=TRUE, "FANS"=TRUE} ("POWERA")
        # "Initialize the shift-register data, here.\n(data names are defined by what you wire into the bundle function)"
        n728 = local write "POWERB"(w1299) -> ()
        n729 = local write "POWERA"(w1299) -> ()
        n730 = local write "POWERC"(w1299) -> ()
        n731 = local write "POWERD"(w1299) -> ()
        n732 = property on="EEV Limit" class="DigNum (strict)"("NumText.BG Color"=w1298) -> ()  [unwired: 2 in, 2 out]
        n733 = property on="Thermal Limit" class="DigNum (strict)"("NumText.BG Color"=w1298) -> ()  [unwired: 2 in, 2 out]
        n734 = call <vilib>:"Add State(s) to Queue__jki_lib_state_machine.vi"("State(s) in (\"\")"=w1303) -> ("States Out"=w1302:string)  [unwired: 14 in]
      }
      frame "UI: Update" {
        w1313 = enum16{"Reset", "Read", "Count Up"}."Read" ("Mode")
        w1324 = T5 {"UE"=FALSE, "LE"=FALSE, "COMP"=FALSE, "FANS"=FALSE} ("POWER 2")
        # "Update User Interface with processed Data"
        n735 = Unbundle By Name(w1323) -> ("Q Element.Serial Data A"=w1322:string[][])
        n736 = Unbundle By Name(w1323) -> ("Q Element.Serial Data C"=w1317:string[][])
        n737 = local read "ComA"() -> (w1308:bool)
        n738 = local read "ComB"() -> (w1305:bool)
        n739 = local read "ComC"() -> (w1306:bool)
        n740 = local read "ComD"() -> (w1307:bool)
        n741 = Unbundle By Name(w1323) -> ("Q Element.Serial Data B"=w1319:string[][])
        n742 = Unbundle By Name(w1323) -> ("Q Element.Serial Data D"=w1316:string[][])
        n743 = Compound Arithmetic op=OR(w1308, w1305, w1306, w1307) -> (w1304:bool)
        n744 = case shown="True" w1304 {
          frame False {
          }
          frame True {
            n745 = local read "Test Started"() -> (w1372:bool)
            n746 = Not(x=w1372) -> (.not. x?=w1373:bool)
            n747 = property on="Start Test" class="Bool (strict)"("Visible"=w1373) -> ()  [unwired: 2 in, 2 out]
          }
        }
        n748 = Transpose 2D Array(2D array=w1322) -> (transposed array=w1321:string[][])
        n749 = Transpose 2D Array(2D array=w1319) -> (transposed array=w1320:string[][])
        n750 = Transpose 2D Array(2D array=w1316) -> (transposed array=w1315:string[][])
        n751 = Transpose 2D Array(2D array=w1317) -> (transposed array=w1318:string[][])
        n752 = for {
          tunnel: w1318 -> [w1381]
          tunnel: string[] ["UpperElement", "LowerElement", "Compressor", "Fan"] ("Header") -> [w1380] mode=indexing
          tunnel: [w1378] -> w1344 mode=indexing
          n753 = call "Array_Search_For_Num.vi"("N Rows of Data"=w1381, "Title?"=w1380) -> ("number"=w1379:dbl)  [unwired: 12 in, 1 out]
          n754 = Greater Than 0?(x=w1379) -> (x > 0?=w1378:bool)
        }
        n755 = for {
          tunnel: w1315 -> [w1377]
          tunnel: string[] ["UpperElement", "LowerElement", "Compressor", "Fan"] ("Header") -> [w1376] mode=indexing
          tunnel: [w1374] -> w1327 mode=indexing
          n756 = call "Array_Search_For_Num.vi"("N Rows of Data"=w1377, "Title?"=w1376) -> ("number"=w1375:dbl)  [unwired: 12 in, 1 out]
          n757 = Greater Than 0?(x=w1375) -> (x > 0?=w1374:bool)
        }
        n758 = for {
          tunnel: w1321 -> [w1389]
          tunnel: string[] ["UpperElement", "LowerElement", "Compressor", "Fan"] ("Header") -> [w1388] mode=indexing
          tunnel: [w1386] -> w1366 mode=indexing
          n759 = call "Array_Search_For_Num.vi"("N Rows of Data"=w1389, "Title?"=w1388) -> ("number"=w1387:dbl)  [unwired: 12 in, 1 out]
          n760 = Greater Than 0?(x=w1387) -> (x > 0?=w1386:bool)
        }
        n761 = for {
          tunnel: w1320 -> [w1385]
          tunnel: string[] ["UpperElement", "LowerElement", "Compressor", "Fan"] ("Header") -> [w1384] mode=indexing
          tunnel: [w1382] -> w1349 mode=indexing
          n762 = call "Array_Search_For_Num.vi"("N Rows of Data"=w1385, "Title?"=w1384) -> ("number"=w1383:dbl)  [unwired: 12 in, 1 out]
          n763 = Greater Than 0?(x=w1383) -> (x > 0?=w1382:bool)
        }
        n764 = Index Array(array=w1344, index #1=0 ("index"), index #2=1 ("index"), index #3=2 ("index"), index #4=3 ("index")) -> (element #1=w1342:bool, element #2=w1340:bool, element #3=w1338:bool, element #4=w1336:bool)
        n765 = Index Array(array=w1327, index #1=0 ("index"), index #2=1 ("index"), index #3=2 ("index"), index #4=3 ("index")) -> (element #1=w1329:bool, element #2=w1331:bool, element #3=w1333:bool, element #4=w1335:bool)
        n766 = Index Array(array=w1366, index #1=0 ("index"), index #2=1 ("index"), index #3=2 ("index"), index #4=3 ("index")) -> (element #1=w1364:bool, element #2=w1362:bool, element #3=w1360:bool, element #4=w1358:bool)
        n767 = Index Array(array=w1349, index #1=0 ("index"), index #2=1 ("index"), index #3=2 ("index"), index #4=3 ("index")) -> (element #1=w1351:bool, element #2=w1353:bool, element #3=w1355:bool, element #4=w1357:bool)
        n768 = Bundle By Name(cluster=w1324, "UE"=w1342, "LE"=w1340, "COMP"=w1338, "FANS"=w1336) -> (→"POWERC":T5)
        n769 = Bundle By Name(cluster=w1324, "UE"=w1329, "LE"=w1331, "COMP"=w1333, "FANS"=w1335) -> (→"POWERD":T5)
        n770 = Bundle By Name(cluster=w1324, "UE"=w1364, "LE"=w1362, "COMP"=w1360, "FANS"=w1358) -> (→"POWERA":T5)
        n771 = Bundle By Name(cluster=w1324, "UE"=w1351, "LE"=w1353, "COMP"=w1355, "FANS"=w1357) -> (→"POWERB":T5)
        n772 = call "String_in_Reference.vi"() -> ("String Out"=→"Status Message":string)  [unwired: 19 in]
        n773 = call "Counter - Save C.vi"("Mode"=w1313) -> ("Counter"=→"Count C":dbl)  [unwired: 10 in]
        n774 = call "Counter - Save A.vi"("Mode"=w1313) -> ("Counter"=→"Count A":dbl)  [unwired: 10 in]
        n775 = call "Counter - Save B.vi"("Mode"=w1313) -> ("Counter"=→"Count B":dbl)  [unwired: 10 in]
        n776 = call "Counter - Save D.vi"("Mode"=w1313) -> ("Counter"=→"Count D":dbl)  [unwired: 10 in]
        n777 = call <vilib>:"Add State(s) to Queue__jki_lib_state_machine.vi"("State(s) in (\"\")"=w1371) -> ("States Out"=w1370:string)  [unwired: 14 in]
      }
      frame "------ DATA ------" {
        # "Do not put any code in this frame.\n(It is a separator no-op. You can make a copy of this frame to create a new Data frame)"
        n778 = call <vilib>:"Add State(s) to Queue__jki_lib_state_machine.vi"("State(s) in (\"\")"=w1393) -> ("States Out"=w1392:string)  [unwired: 14 in]
      }
      frame "Data: Initialize" {
        w1394 = T20 {"Alarm A"=FALSE, "Current Draw(A)"=2, "ComA"=TRUE, "POWER"={"UE"=FALSE, "LE"=FALSE, "COMP"=FALSE, "FANS"=FALSE}}  # RLT TankD
        w1395 = T20 {"Alarm A"=FALSE, "Current Draw(A)"=2, "ComA"=TRUE, "POWER"={"UE"=FALSE, "LE"=FALSE, "COMP"=FALSE, "FANS"=FALSE}}  # RLT Tank C
        w1396 = T20 {"Alarm A"=FALSE, "Current Draw(A)"=2, "ComA"=TRUE, "POWER"={"UE"=FALSE, "LE"=FALSE, "COMP"=FALSE, "FANS"=FALSE}}  # RLT Tank B
        w1397 = T20 {"Alarm A"=FALSE, "Current Draw(A)"=2, "ComA"=TRUE, "POWER"={"UE"=FALSE, "LE"=FALSE, "COMP"=FALSE, "FANS"=FALSE}}  # RLT Tank A
        w1398 = enum16{"Reset", "Read", "Count Up"}."Reset" ("Mode")
        w1400 = string[][] []  # D Data Array
        w1401 = string[][] []  # C Data Array
        w1402 = string[][] []  # B Data Array
        w1403 = string[][] []  # A Data Array
        w1399 = T21 {"MW100 Data"=[], "Serial Data A"=[], "Serial Data B"=[], "Serial Data C"=[], "Serial Data D"=[], "Agilent Output Data"=[]}  # Q Element
        n779 = call <vilib>:"Add State(s) to Queue__jki_lib_state_machine.vi"("State(s) in (\"\")"=w1408) -> ("States Out"=w1407:string)  [unwired: 14 in]
        n780 = Bundle(cluster=w1405, "Q Element"=w1399, "A Data Array"=w1403, "B Data Array"=w1402, "C Data Array"=w1401, "D Data Array"=w1400, "RLT Tank A"=w1397, "RLT Tank B"=w1396, "RLT Tank C"=w1395, "RLT TankD"=w1394) -> (w1404:T22)
        n781 = call "Counter - Save A.vi"("Mode"=w1398) -> ()  [unwired: 10 in, 1 out]
        n782 = call "Counter - Save B.vi"("Mode"=w1398) -> ()  [unwired: 10 in, 1 out]
        n783 = call "Counter - Save C.vi"("Mode"=w1398) -> ()  [unwired: 10 in, 1 out]
        n784 = call "Counter - Save D.vi"("Mode"=w1398) -> ()  [unwired: 10 in, 1 out]
      }
      frame "Data: DeQueue" {
        # "Your code here.\n(You can make a copy of, or modify, this frame)"
        n785 = flat-sequence {
          tunnel: [w1418] -> w1409
          frame #0 {
            n786 = while {
              stop <- w1416 stop-if-true
              n787 = local read "# elements in queue"() -> (w1417:i32)
              n788 = Wait (ms)(milliseconds to wait=u32 500) -> ()  [unwired: 1 out]
              n789 = Greater Than 0?(x=w1417) -> (x > 0?=w1416:bool)
            }
          }
          frame #1 {
            n790 = local read "DataQ"() -> (w1419:refnum<queue>)
            n791 = Dequeue Element(queue=w1419) -> (element=w1418:T21)  [unwired: 2 in, 3 out]
          }
        }
        n792 = Bundle By Name(cluster=w1411, "Q Element"=w1409) -> (w1410:T22)
        n793 = call <vilib>:"Add State(s) to Queue__jki_lib_state_machine.vi"("State(s) in (\"\")"=w1414) -> ("States Out"=w1413:string)  [unwired: 14 in]
      }
      frame "Data: Process" {
        # "Process Data Steps.\nPuts the gathered data into arrays to be saved."
        n794 = call <vilib>:"Add State(s) to Queue__jki_lib_state_machine.vi"("State(s) in Front (\"\")"="Data: Process MW100\nData: Process Agilent\nData: Process Check Limits\nData: Process Serial\nData: Process Time" ("State(s) in Front (\"\")"), "State(s) in (\"\")"=w1424) -> ("States Out"=w1423:string)  [unwired: 13 in]
      }
      frame "Data: Process MW100" {
        w1446 = string[] ["011", "012", "013", "014", "015", "016", "017", "018", "019", "020", "021", "022", "023", "024", "025", "026", "027", "028", "029", "030", "031", "032", "033", "034", "035", "036", "A001", "A002", "A003", "A004", "A005", "A006", "A007", "A008", "A009", "A010"] ("deleted portion")
        # "Your code here.\n(You can make a copy of, or modify, this frame)"
        n795 = Unbundle By Name(w1439) -> ("Q Element.MW100 Data"=w1427:dbl[])
        n796 = Index Array(array=w1427, index=16) -> (element=→"Tc_down":dbl)
        n797 = local read "Station A Channels, MW100"() -> (w1443:string[])
        n798 = local read "Station D Channels, MW100"() -> (w1441:string[])
        n799 = local read "Station A Labels, MW100"() -> (w1433:string[])
        n800 = local read "Station B Channels, MW100"() -> (w1440:string[])
        n801 = local read "Station B Labels, MW100"() -> (w1432:string[])
        n802 = local read "Station C Channels, MW100"() -> (w1442:string[])
        n803 = local read "Station D Labels, MW100"() -> (w1430:string[])
        n804 = local read "Station C Labels, MW100"() -> (w1431:string[])
        n805 = Array Size(array=w1446) -> (size(s)=w1445:i32)
        n806 = Number To Fractional String(number=w1427) -> (F-format string=w1447:string[])  [unwired: 3 in]
        n807 = Initialize Array("DUMMYVAL" ("String"), 2 ("dimension size"), w1445) -> (w1450:string[][])
        n808 = Replace Array Subset(array=w1450, new element #1=w1446, index (row) #1=0 ("index"), new element #2=w1447, index (row) #2=1 ("index")) -> (w1428:string[][])  [unwired: 2 in]
        n809 = call "HEWH MW100 Cut Unneeded Data.vi"("MW100 Data In"=w1428) -> ("MW100 Data Out"=w1429:string[][])  [unwired: 10 in]
        n810 = for {
          tunnel: w1429 -> [w1478]
          tunnel: w1443 -> [w1477] mode=indexing
          tunnel: [w1474] -> w1437 mode=indexing
          tunnel: w1433 -> [w1473] mode=indexing
          n811 = call "Array_Search_For_Num.vi"("N Rows of Data"=w1478, "Title?"=w1477) -> ("number"=w1476:dbl)  [unwired: 12 in, 1 out]
          n812 = Number To Fractional String(number=w1476) -> (F-format string=w1475:string)  [unwired: 3 in]
          n813 = Build Array(w1473, w1475) -> (w1474:string[])
        }
        n814 = for {
          tunnel: w1429 -> [w1472]
          tunnel: w1440 -> [w1471] mode=indexing
          tunnel: [w1468] -> w1436 mode=indexing
          tunnel: w1432 -> [w1467] mode=indexing
          n815 = call "Array_Search_For_Num.vi"("N Rows of Data"=w1472, "Title?"=w1471) -> ("number"=w1470:dbl)  [unwired: 12 in, 1 out]
          n816 = Number To Fractional String(number=w1470) -> (F-format string=w1469:string)  [unwired: 3 in]
          n817 = Build Array(w1467, w1469) -> (w1468:string[])
        }
        n818 = for {
          tunnel: w1429 -> [w1460]
          tunnel: w1441 -> [w1459] mode=indexing
          tunnel: [w1456] -> w1434 mode=indexing
          tunnel: w1430 -> [w1455] mode=indexing
          n819 = call "Array_Search_For_Num.vi"("N Rows of Data"=w1460, "Title?"=w1459) -> ("number"=w1458:dbl)  [unwired: 12 in, 1 out]
          n820 = Number To Fractional String(number=w1458) -> (F-format string=w1457:string)  [unwired: 3 in]
          n821 = Build Array(w1455, w1457) -> (w1456:string[])
        }
        n822 = for {
          tunnel: w1429 -> [w1466]
          tunnel: w1442 -> [w1465] mode=indexing
          tunnel: [w1462] -> w1435 mode=indexing
          tunnel: w1431 -> [w1461] mode=indexing
          n823 = call "Array_Search_For_Num.vi"("N Rows of Data"=w1466, "Title?"=w1465) -> ("number"=w1464:dbl)  [unwired: 12 in, 1 out]
          n824 = Number To Fractional String(number=w1464) -> (F-format string=w1463:string)  [unwired: 3 in]
          n825 = Build Array(w1461, w1463) -> (w1462:string[])
        }
        n826 = call <vilib>:"Add State(s) to Queue__jki_lib_state_machine.vi"("State(s) in (\"\")"=w1454) -> ("States Out"=w1453:string)  [unwired: 14 in]
        n827 = Bundle By Name(cluster=w1439, "A Data Array"=w1437, "B Data Array"=w1436, "C Data Array"=w1435, "D Data Array"=w1434) -> (w1438:T22)
      }
      frame "Data: Process Agilent" {
        # "Sort our Agilent data for saving."
        n828 = Unbundle By Name(w1495) -> ("Q Element.Agilent Output Data"=w1496:dbl[], "A Data Array"=w1493:string[][], "B Data Array"=w1489:string[][], "C Data Array"=w1484:string[][], "D Data Array"=w1479:string[][])
        n829 = local read "Station A Labels, Agilent"() -> (w1491:string[])
        n830 = local read "Station B Labels, Agilent"() -> (w1487:string[])
        n831 = local read "Station C Labels, Agilent"() -> (w1481:string[])
        n832 = local read "Station D Labels, Agilent"() -> (w1480:string[])
        n833 = call "HEWH RLT Process Agilent Data.vi"("Data Array"=w1493, "Labels, Agilent"=w1491, "Agilent Data"=w1496) -> ("Appended Data Array"=w1492:string[][], "Data array w/ subset deleted"=w1490:dbl[])  [unwired: 11 in]
        n834 = call "HEWH RLT Process Agilent Data.vi"("Data Array"=w1489, "Labels, Agilent"=w1487, "Agilent Data"=w1490) -> ("Appended Data Array"=w1488:string[][], "Data array w/ subset deleted"=w1486:dbl[])  [unwired: 11 in]
        n835 = call "HEWH RLT Process Agilent Data.vi"("Data Array"=w1484, "Labels, Agilent"=w1481, "Agilent Data"=w1486) -> ("Appended Data Array"=w1483:string[][], "Data array w/ subset deleted"=w1485:dbl[])  [unwired: 11 in]
        n836 = call "HEWH RLT Process Agilent Data.vi"("Data Array"=w1479, "Labels, Agilent"=w1480, "Agilent Data"=w1485) -> ("Appended Data Array"=w1482:string[][])  [unwired: 11 in, 1 out]
        n837 = call <vilib>:"Add State(s) to Queue__jki_lib_state_machine.vi"("State(s) in (\"\")"=w1499) -> ("States Out"=w1498:string)  [unwired: 14 in]
        n838 = Bundle By Name(cluster=w1495, "A Data Array"=w1492, "B Data Array"=w1488, "C Data Array"=w1483, "D Data Array"=w1482) -> (w1494:T22)
      }
      frame "Data: Process Check Limits" {
        w1508 = 0  # Gallons position,
        # "Latch Over Temp Alarms On"
        # "Check all data gathered in current records for themal limit. Exclude Gallons!"
        n839 = Unbundle By Name(w1550) -> ("A Data Array"=w1549:string[][], "B Data Array"=w1540:string[][], "C Data Array"=w1536:string[][], "D Data Array"=w1530:string[][])
        n840 = Index Array(array=w1530, index (col)=1 ("disabled index (col)")) -> (element=w1510:string[])  [unwired: 1 in]
        n841 = Index Array(array=w1540, index (col)=1 ("disabled index (col)")) -> (element=w1513:string[])  [unwired: 1 in]
        n842 = Index Array(array=w1536, index (col)=1 ("disabled index (col)")) -> (element=w1512:string[])  [unwired: 1 in]
        n843 = Index Array(array=w1549, index (col)=1 ("disabled index (col)")) -> (element=w1516:string[])  [unwired: 1 in]
        n844 = Delete From Array(array=w1516, index=w1508) -> (array with subset deleted=w1515:string[])  [unwired: 1 in, 1 out]
        n845 = Delete From Array(array=w1513, index=w1508) -> (array with subset deleted=w1514:string[])  [unwired: 1 in, 1 out]
        n846 = Delete From Array(array=w1510, index=w1508) -> (array with subset deleted=w1509:string[])  [unwired: 1 in, 1 out]
        n847 = Delete From Array(array=w1512, index=w1508) -> (array with subset deleted=w1511:string[])  [unwired: 1 in, 1 out]
        n848 = Fract/Exp String To Number(string=w1509) -> (number=w1533:dbl[])  [unwired: 3 in, 1 out]
        n849 = Fract/Exp String To Number(string=w1515) -> (number=w1547:dbl[])  [unwired: 3 in, 1 out]
        n850 = Fract/Exp String To Number(string=w1514) -> (number=w1542:dbl[])  [unwired: 3 in, 1 out]
        n851 = Fract/Exp String To Number(string=w1511) -> (number=w1538:dbl[])  [unwired: 3 in, 1 out]
        n852 = Greater Or Equal?(x=w1538, y="Thermal Limit") -> (x >= y?=w1537:bool[])
        n853 = Greater Or Equal?(x=w1533, y="Thermal Limit") -> (x >= y?=w1534:bool[])
        n854 = local read "No Draw D"() -> (w1500:bool)
        n855 = local read "No Draw A"() -> (w1506:bool)
        n856 = Greater Or Equal?(x=w1547, y="Thermal Limit") -> (x >= y?=w1546:bool[])
        n857 = Greater Or Equal?(x=w1542, y="Thermal Limit") -> (x >= y?=w1543:bool[])
        n858 = local read "Alarm A"() -> (w1529:bool)
        n859 = local read "No Draw C"() -> (w1502:bool)
        n860 = local read "ComA"() -> (w1526:bool)
        n861 = Or Array Elements(Boolean array=w1537) -> (logical OR=w1528:bool)
        n862 = local read "Alarm D"() -> (w1519:bool)
        n863 = local read "No Draw B"() -> (w1504:bool)
        n864 = Or Array Elements(Boolean array=w1534) -> (logical OR=w1535:bool)
        n865 = local read "Alarm C"() -> (w1521:bool)
        n866 = local read "ComD"() -> (w1518:bool)
        n867 = local read "ComC"() -> (w1520:bool)
        n868 = Or Array Elements(Boolean array=w1546) -> (logical OR=w1545:bool)
        n869 = Or Array Elements(Boolean array=w1543) -> (logical OR=w1544:bool)
        n870 = local read "Alarm B"() -> (w1524:bool)
        n871 = local read "ComB"() -> (w1523:bool)
        n872 = Compound Arithmetic op=AND(invert w1521, w1520) -> (w1522:bool)
        n873 = Compound Arithmetic op=AND(invert w1529, w1526) -> (w1527:bool)
        n874 = Compound Arithmetic op=AND(invert w1519, w1518) -> (w1517:bool)
        n875 = Or(x=w1506, y=w1545) -> (x .or. y?=w1507:bool)
        n876 = Compound Arithmetic op=AND(invert w1524, w1523) -> (w1525:bool)
        n877 = Or(x=w1504, y=w1544) -> (x .or. y?=w1505:bool)
        n878 = Or(x=w1502, y=w1528) -> (x .or. y?=w1503:bool)
        n879 = Or(x=w1535, y=w1500) -> (x .or. y?=w1501:bool)
        n880 = case shown="True" w1527 {
          tunnel: w1507 -> [_ w1560]
          frame False {
          }
          frame True {
            n881 = case shown="True" w1560 {
              frame False {
              }
              frame True {
                n882 = property on="Thermal Limit" class="DigNum (strict)"("NumText.BG Color"=u32 16711680 ("Color Box")) -> ()  [unwired: 2 in, 2 out]
              }
            }
            "Alarm A" <- w1560
          }
        }
        n883 = case shown="True" w1525 {
          tunnel: w1505 -> [_ w1558]
          frame False {
          }
          frame True {
            n884 = case shown="True" w1558 {
              frame False {
              }
              frame True {
                n885 = property on="Thermal Limit" class="DigNum (strict)"("NumText.BG Color"=u32 16711680 ("Color Box")) -> ()  [unwired: 2 in, 2 out]
              }
            }
            "Alarm B" <- w1558
          }
        }
        n886 = case shown="True" w1522 {
          tunnel: w1503 -> [_ w1556]
          frame False {
          }
          frame True {
            n887 = case shown="True" w1556 {
              frame False {
              }
              frame True {
                n888 = property on="Thermal Limit" class="DigNum (strict)"("NumText.BG Color"=u32 16711680 ("Color Box")) -> ()  [unwired: 2 in, 2 out]
              }
            }
            "Alarm C" <- w1556
          }
        }
        n889 = case shown="True" w1517 {
          tunnel: w1501 -> [_ w1554]
          frame False {
          }
          frame True {
            n890 = case shown="True" w1554 {
              frame False {
              }
              frame True {
                n891 = property on="Thermal Limit" class="DigNum (strict)"("NumText.BG Color"=u32 16711680 ("Color Box")) -> ()  [unwired: 2 in, 2 out]
              }
            }
            "Alarm D" <- w1554
          }
        }
        n892 = call <vilib>:"Add State(s) to Queue__jki_lib_state_machine.vi"("State(s) in (\"\")"=w1553) -> ("States Out"=w1552:string)  [unwired: 14 in]
      }
      frame "Data: Process Serial" {
        # "Sort our Agilent data for saving."
        n893 = Unbundle By Name(w1600) -> ("A Data Array"=w1595:string[][], "Q Element.Serial Data A"=w1590:string[][], "B Data Array"=w1596:string[][], "Q Element.Serial Data B"=w1564:string[][], "C Data Array"=w1597:string[][], "Q Element.Serial Data C"=w1563:string[][], "D Data Array"=w1598:string[][], "Q Element.Serial Data D"=w1562:string[][])
        n894 = local read "Alarm A"() -> (w1577:bool)
        n895 = local read "ComA"() -> (w1576:bool)
        n896 = local read "Alarm C"() -> (w1569:bool)
        n897 = local read "Alarm B"() -> (w1572:bool)
        n898 = local read "ComB"() -> (w1571:bool)
        n899 = local read "Alarm D"() -> (w1567:bool)
        n900 = local read "ComC"() -> (w1568:bool)
        n901 = local read "ComD"() -> (w1566:bool)
        n902 = call "Array_Search_For_Num.vi"("N Rows of Data"=w1590, "Title?"="EEV") -> ("number"=w1588:dbl)  [unwired: 12 in, 1 out]
        n903 = Compound Arithmetic op=AND(w1576, invert w1577) -> (w1575:bool)
        n904 = call "Array_Search_For_Num.vi"("N Rows of Data"=w1562, "Title?"="EEV") -> ("number"=w1580:dbl)  [unwired: 12 in, 1 out]
        n905 = call "Array_Search_For_Num.vi"("N Rows of Data"=w1564, "Title?"="EEV") -> ("number"=w1586:dbl)  [unwired: 12 in, 1 out]
        n906 = call "Array_Search_For_Num.vi"("N Rows of Data"=w1563, "Title?"="EEV") -> ("number"=w1583:dbl)  [unwired: 12 in, 1 out]
        n907 = Greater Or Equal?(x=w1588, y="EEV Limit") -> (x >= y?=w1587:bool)
        n908 = Greater Or Equal?(x=w1580, y="EEV Limit") -> (x >= y?=w1581:bool)
        n909 = Greater Or Equal?(x=w1586, y="EEV Limit") -> (x >= y?=w1574:bool)
        n910 = Compound Arithmetic op=AND(w1566, invert w1567) -> (w1565:bool)
        n911 = Compound Arithmetic op=AND(w1568, invert w1569) -> (w1570:bool)
        n912 = Greater Or Equal?(x=w1583, y="EEV Limit") -> (x >= y?=w1582:bool)
        n913 = Compound Arithmetic op=AND(w1571, invert w1572) -> (w1573:bool)
        n914 = case shown="True" w1575 {
          tunnel: w1587 -> [_ w1610]
          frame False {
          }
          frame True {
            n915 = local write "Alarm A"(w1610) -> ()
            n916 = case shown="True" w1610 {
              frame False {
              }
              frame True {
                n917 = property on="EEV Limit" class="DigNum (strict)"("NumText.BG Color"=u32 16711680 ("Color Box")) -> ()  [unwired: 2 in, 2 out]
              }
            }
          }
        }
        n918 = case shown="True" w1573 {
          tunnel: w1574 -> [_ w1608]
          frame False {
          }
          frame True {
            n919 = local write "Alarm B"(w1608) -> ()
            n920 = case shown="True" w1608 {
              frame False {
              }
              frame True {
                n921 = property on="EEV Limit" class="DigNum (strict)"("NumText.BG Color"=u32 16711680 ("Color Box")) -> ()  [unwired: 2 in, 2 out]
              }
            }
          }
        }
        n922 = case shown="True" w1570 {
          tunnel: w1582 -> [_ w1606]
          frame False {
          }
          frame True {
            n923 = local write "Alarm C"(w1606) -> ()
            n924 = case shown="True" w1606 {
              frame False {
              }
              frame True {
                n925 = property on="EEV Limit" class="DigNum (strict)"("NumText.BG Color"=u32 16711680 ("Color Box")) -> ()  [unwired: 2 in, 2 out]
              }
            }
          }
        }
        n926 = case shown="True" w1565 {
          tunnel: w1581 -> [_ w1604]
          frame False {
          }
          frame True {
            n927 = local write "Alarm D"(w1604) -> ()
            n928 = case shown="True" w1604 {
              frame False {
              }
              frame True {
                n929 = property on="EEV Limit" class="DigNum (strict)"("NumText.BG Color"=u32 16711680 ("Color Box")) -> ()  [unwired: 2 in, 2 out]
              }
            }
          }
        }
        n930 = Build Array (concatenate)(w1597, w1563) -> (w1592:string[][])
        n931 = Build Array (concatenate)(w1598, w1562) -> (w1591:string[][])
        n932 = Build Array (concatenate)(w1596, w1564) -> (w1593:string[][])
        n933 = Build Array (concatenate)(w1595, w1590) -> (w1594:string[][])
        n934 = call <vilib>:"Add State(s) to Queue__jki_lib_state_machine.vi"("State(s) in (\"\")"=w1603) -> ("States Out"=w1602:string)  [unwired: 14 in]
        n935 = Bundle By Name(cluster=w1600, "A Data Array"=w1594, "B Data Array"=w1593, "C Data Array"=w1592, "D Data Array"=w1591) -> (w1599:T22)
      }
      frame "Data: Process Time" {
        # "Sort our Agilent data for saving."
        n936 = Unbundle By Name(w1612) -> ("A Data Array"=w1620:string[][], "B Data Array"=w1619:string[][], "C Data Array"=w1618:string[][], "D Data Array"=w1617:string[][])
        n937 = call "E-Time.vi"() -> ("Elapsed Time (sec)"=w1623:dbl)  [unwired: 9 in, 2 out]
        "Elapsed Time" <- w1623
        n938 = Number To Fractional String(number=w1623) -> (F-format string=w1626:string)  [unwired: 3 in]
        n939 = Build Array("Elapsed Time", w1626) -> (w1622:string[])
        n940 = Build Array(w1622) -> (w1621:string[][])
        n941 = Build Array (concatenate)(w1621, w1619) -> (w1614:string[][])
        n942 = Build Array (concatenate)(w1621, w1620) -> (w1613:string[][])
        n943 = Build Array (concatenate)(w1621, w1618) -> (w1615:string[][])
        n944 = Build Array (concatenate)(w1621, w1617) -> (w1616:string[][])
        n945 = call <vilib>:"Add State(s) to Queue__jki_lib_state_machine.vi"("State(s) in (\"\")"=w1629) -> ("States Out"=w1628:string)  [unwired: 14 in]
        n946 = Bundle By Name(cluster=w1612, "A Data Array"=w1613, "B Data Array"=w1614, "C Data Array"=w1615, "D Data Array"=w1616) -> (w1625:T22)
      }
      frame "Data: Save" {
        # "Your code here.\n(You can make a copy of, or modify, this frame)"
        n947 = Unbundle By Name(w1650) -> ("A Data Array"=w1649:string[][], "B Data Array"=w1648:string[][], "C Data Array"=w1647:string[][], "D Data Array"=w1646:string[][])
        "A Data Array" <- w1649
        "B Data Array" <- w1648
        "C Data Array" <- w1647
        "D Data Array" <- w1646
        n948 = Transpose 2D Array(2D array=w1649) -> (transposed array=w1644:string[][])
        n949 = Transpose 2D Array(2D array=w1648) -> (transposed array=w1641:string[][])
        n950 = Transpose 2D Array(2D array=w1647) -> (transposed array=w1639:string[][])
        n951 = Transpose 2D Array(2D array=w1646) -> (transposed array=w1636:string[][])
        n952 = local read "FileNameB"() -> (w1642:path)
        n953 = local read "FileNameD"() -> (w1635:path)
        n954 = local read "FileNameA"() -> (w1645:path)
        n955 = local read "FileNameC"() -> (w1640:path)
        n956 = local read "ComB"() -> (w1632:bool)
        n957 = local read "ComD"() -> (w1630:bool)
        n958 = local read "ComA"() -> (w1633:bool)
        n959 = local read "ComC"() -> (w1631:bool)
        n960 = call "HEWH RLT Save Data.vi"("file path (dialog if empty)"=w1645, "Data Array"=w1644, "index"=enum16{"A", "B", "C", "D"}."A", "Enable Save"=w1633) -> ()  [unwired: 12 in]
        n961 = call "HEWH RLT Save Data.vi"("file path (dialog if empty)"=w1642, "Data Array"=w1641, "index"=enum16{"A", "B", "C", "D"}."B", "Enable Save"=w1632) -> ()  [unwired: 12 in]
        n962 = call "HEWH RLT Save Data.vi"("file path (dialog if empty)"=w1640, "Data Array"=w1639, "index"=enum16{"A", "B", "C", "D"}."C", "Enable Save"=w1631) -> ()  [unwired: 12 in]
        n963 = call "HEWH RLT Save Data.vi"("file path (dialog if empty)"=w1635, "Data Array"=w1636, "index"=enum16{"A", "B", "C", "D"}."D", "Enable Save"=w1630) -> ()  [unwired: 12 in]
        n964 = call <vilib>:"Add State(s) to Queue__jki_lib_state_machine.vi"("State(s) in (\"\")"=w1653) -> ("States Out"=w1652:string)  [unwired: 14 in]
      }
    }
  }
